vi "DB - [Setup].[Item] (Part Details).vi"(0 "connection reference":T14, 1 "DB Connection":T7={"Open"=TRUE, "Close"=TRUE}, 2 "DB - Setup Item Enum":T13=enum."INSERT [Setup].[Item]", 5 "DB.Schema.Table Array":string[](array[string]), 7 "Search Parameters":string, 9 "Transaction":T5, 11 "error in (no error)":errorcluster, 12 "DB Refnums":T6, 13 "OrderNo":string="101", 14 "DB Refnums II":T4) -> (3 "[IsMandatory] Ordered":string[](array[string]), 4 "connection reference":T14, 6 "1D Results":string[](array[string]), 8 "2D Results":string[][](array[string])=[["Production", "OperationNo1"], ["Production", "Qty1"], ["Production", "NCRNo1"], ["Production", "CustomerID1"], ["Production", "Customer1"], ["Production", "Project1"], ["Production", "SalesOrderNo1"], ["Production", "SalesOrderItemNo1"], ["Production", "MaterialNo1"], ["Production", "MaterialRev1"], ["Production", "MaterialDesc1"], ["Production", "SerialNos1"], ["Production", "UnitOfQty1"]], 10 "Transaction":T5, 15 "SUMMARY":errorcluster)   [LabVIEW 2020]
uses:
  <vilib>/addons/database/Connection.llb/Conn ObjectReference.ctl
  Control/DB - Setup Item Enum.ctl
  Control/Setup - Part Details - Item Details.ctl
  Control/Combo Box.ctl
  Control/DB - Logon Info.ctl
  Control/DB - OpenClose.ctl
  Control/DB - Refnums.ctl
  Control/Transaction Cluster.ctl
  Control/DB - Refnums II.ctl
  Control/Execute - Info.ctl
  Control/DB - [Setup].[Header] ColNames.ctl
  Control/DB - [TransactionNo],[OrderNo].ctl
  Variables/Global SRTRS.vi
  <vilib>/addons/database/Connection.llb/DB Tools Open Connec (String).vi
  <vilib>/addons/database/Connection.llb/Conn Execute.vi
  <vilib>/addons/database/Recordset.llb/Rec Fetch Recordset Data (R).vi
  <vilib>/addons/database/Recordset.llb/Rec Destroy - Connection.vi
  <vilib>/addons/database/Recordset.llb/Rec Fetch String Data (R).vi
  <vilib>/addons/database/_DB Variant To Data/Database Variant To Data.xnode
  <vilib>/addons/database/NI_Database_API.lvlib
panel:
  out "CASTed String":string
  out "SQL 1D Array":string[](array[string])
  in  "Results Output":cluster{"Output Set":T1, "Description":string}
  out "Ref error out":errorcluster={"status"=TRUE, "code"=1055, "source"="To More Specific Class in DB - Setup Item (Part Details).vi->Main.vi"}
  in  "Info. (Execute Tab)":T2 caption="Info." {"Variant Allowed (Hold Temp)" format="%.1f"}
  in  "CompactRIO Module Details":i32(listbox)=-1
  in  "Furnace Calibration":T3={"Furnace Serial No"="100", "Last Inspection Date"="2013-12-05", "Next Inspection Due Date"="2014-12-05"} caption="Furnace Details"
  out "Close Error":errorcluster
  out "Spreadsheet String":string[](array[string])
  in  "MCListBox FHS Setup":i32(listbox)=-1 caption="Furnace Heating Sequence"
  out "Refnums error out":errorcluster={"status"=TRUE, "code"=1055, "source"="To More Specific Class in DB - Setup Item (Part Details).vi->Main.vi"}
  in  "Part Details":i32(listbox)=-1
  in  "MCListBox AWPS":i32(listbox)=-1 caption="Additional WPS/Ref MCListBox"
  in  "Login":T8={"PlantID"="4070", "SystemID"="SRSB-2A", "UserID"="100001", "DomainID"="CCC", "LanguageID"="EN", "StationID"=""}
  in  "WPS Details Setup":T9={"WPS/Ref"="WPS5", "Rev"="1", "Hold Temperature"="100", "WPS Details Temperature Units"="°C", "Hold Time (HH:MM)"="1:00", "Inactive"=FALSE} caption="WPS Details"
  in  "Extra WPS":string caption="WPS"
  in  "Extra Rev":string caption="Rev."
  out "SQL 2D":string="Use [SRTRS]\n\nSELECT TOP 1 \n       [SourceTableName]\n      ,[SourceColumnName]\nFROM [Config].[Mapping]\nWHERE [TargetColumnName] = 'UnitOfQty'\n"
  in  "Channel Mapping":T10 caption="Channels Mapping"
  in  "Item Details":T11={"Order No."="102", "Oper. No."="102", "Qty."=1, "NCR No."="102", "NCR Boolean"=FALSE, "Customer No."="102", "Customer Name"="Cust102", "Project"="Proj102", "Sales Order"="SO102", "Item No."="SOI102", "Material"="M102", "Revision"="1", "Material Description"="", "Serial No."="102", "UnitOfQty"="Pallet"} {"Qty." min=1 max=99}
  in  "Notes":string="Hello World"
  in  "Plot":T12
  out "ms":u32
  out "Connection Information":T15={"Connection "="SQL Server 32bit HPEnvy", "Username"="admin", "Password"="admin123"}
  # "ONLY Witten to during LOGON (initialization)"
  # "For SELECT h.[TransactionNo], i.[OrderNo]\n\nSRTRS.Execute.Header\nSRTRS.Execute.Item\nSRTRS.MasterData.OutputSet"
  # "SRTRS.Setup.Header\nSRTRS.Setup.Item\nSRTRS.MasterData.OutputSet"
  # "Login\nItem Details\nWPS Details\nWPS (Extra)\nRev (Extra)\nAddtional WPS\nNotes\nParts Details (MCListBox)"
  # "[SourceTableName]        [SourceColumnName]           [IsMandatory]                 [TargetColumnName]"
  # "Column Hdrs[] are Important \nMust match with SRTRS Main.vi"
  # "Min"
  # "Min"
  # "Thermocouple"
  # "Probe No."
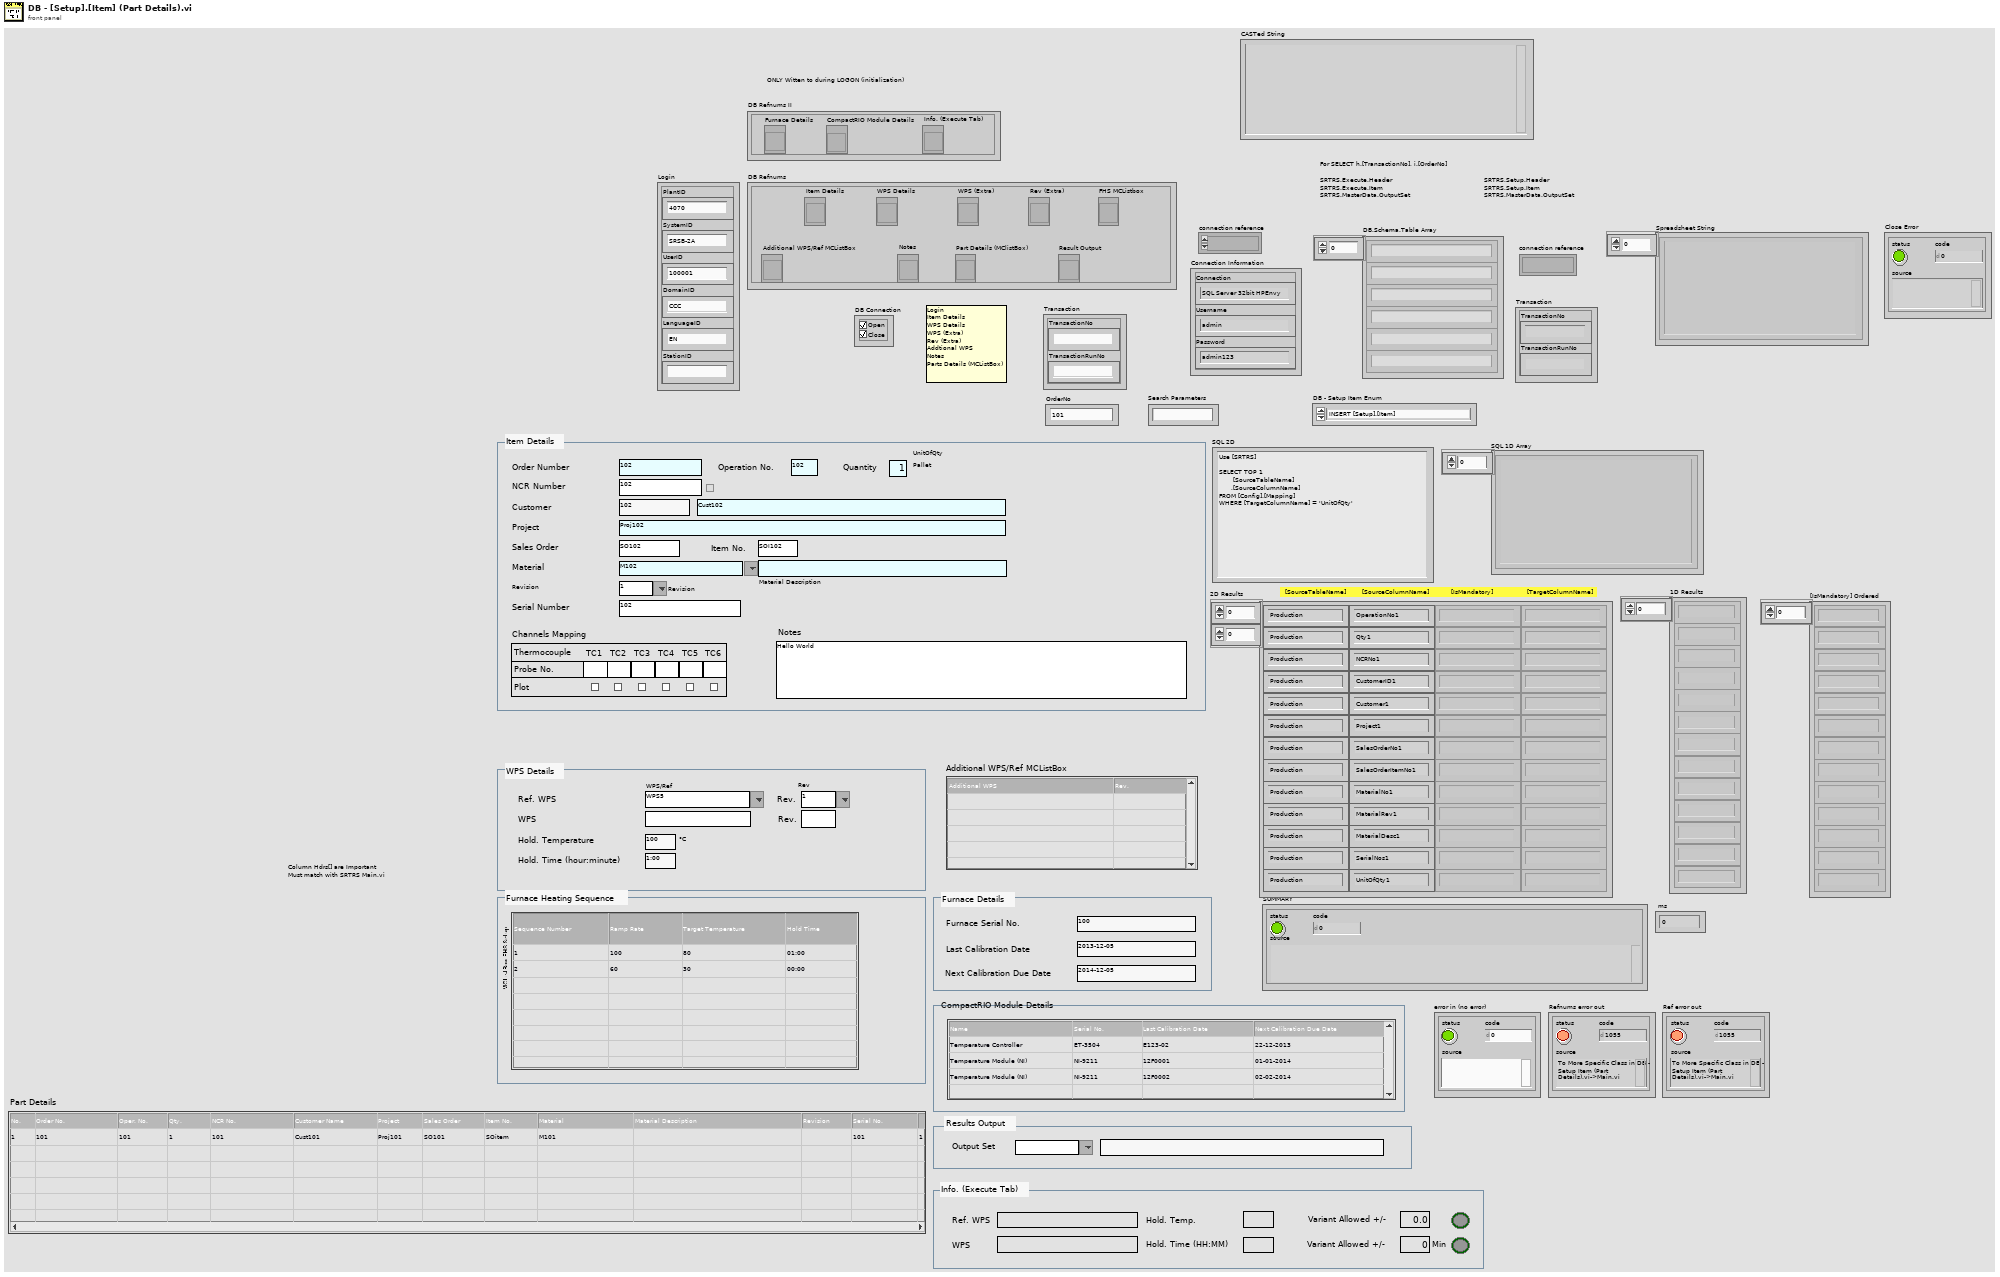
[diagram p1: front panel]
types:
  T1 = typedef "Combo Box.ctl" = string
  T2 = typedef "Execute - Info.ctl" = cluster{"Ref WPS":string, "Hold. Temp.":string, "Info. Temperature Units":string, "Variant Allowed (Hold Temp)":dbl, "Info. Temperature Units 2":string, "Variant Allowed (Hold Temp)":bool, "Hold. Time (hour:minute)":string, "Variant Allowed (Hold Time)":dbl, "Variant Allowed (Hold Time)":bool, "WPS":string}
  T3 = cluster{"Furnace Serial No":string, "Last Inspection Date":string, "Next Inspection Due Date":string}
  T4 = typedef "DB - Refnums II.ctl" = cluster{"Furnace Details":refnum<vi>, "CompactRIO Module Details":refnum<vi>, "Info. (Execute Tab)":refnum<vi>}
  T5 = typedef "Transaction Cluster.ctl" = cluster{"TransactionNo":string, "TransactionRunNo":string}
  T6 = typedef "DB - Refnums.ctl" = cluster{"Item Details":refnum<vi>, "WPS Details":refnum<vi>, "WPS (Extra)":refnum<vi>, "Rev (Extra) ":refnum<vi>, "FHS MCListbox":refnum<vi>, "Additional WPS/Ref MCListBox":refnum<vi>, "Notes":refnum<vi>, "Part Details (MClistBox)":refnum<vi>, "Result Output":refnum<vi>}
  T7 = typedef "DB - OpenClose.ctl" = cluster{"Open":bool, "Close":bool}
  T8 = typedef "DB - Logon Info.ctl" = cluster{"PlantID":string, "SystemID":string, "UserID":string, "DomainID":string, "LanguageID":string, "StationID":string}
  T9 = cluster{"WPS/Ref":T1, "Rev":T1, "Hold Temperature":string, "WPS Details Temperature Units":string, "Hold Time (HH:MM)":string, "Inactive":bool}
  T10 = cluster{"TC1":string, "TC2":string, "TC3":string, "TC4":string, "TC5":string, "TC6":string}
  T11 = typedef "Setup - Part Details - Item Details.ctl" = cluster{"Order No.":string, "Oper. No.":string, "Qty.":i32, "NCR No.":string, "NCR Boolean":bool, "Customer No.":string, "Customer Name":string, "Project":string, "Sales Order":string, "Item No.":string, "Material":string, "Revision":string, "Material Description":string, "Serial No.":string, "UnitOfQty":string}
  T12 = cluster{"TC01Plot":bool, "TC02Plot":bool, "TC03Plot":bool, "TC04Plot":bool, "TC05Plot":bool, "TC06Plot":bool}
  T13 = typedef "DB - Setup Item Enum.ctl" = enum16{"SELECT [Plant],[OrderNo]", "INSERT [Setup].[Header]", "INSERT [Setup].[Item]", "INSERT [Setup].[ProcedureItem]", "SELECT [TransactionNo]", "SELECT [TransactionNo], others", "SELECT [OrderNo]", "SELECT [OrderNo], others", "SELECT h.[TransactionNo], i.[OrderNo]", "SELECT [Setup].[ProcedureItem]", "SELECT [EquipmentxId]"}
  T14 = typedef "NI_Database_API.lvlib/Conn ObjectReference.ctl" = refnum<k1>
  T15 = cluster{"Connection ":string, "Username":string, "Password":string}
  T16 = typedef "Enum - InteractiveMode-SubVIMode.ctl" = enum16{"Interactive", "subVI Mode"}
  T17 = typedef "Connection Information Cluster.ctl" = cluster{"Connection ":string, "Username":string, "Password":string}
  T18 = typedef "DB - DB.Schema.Table.ctl" = cluster{"DB":string, "Schema":string, "Table":string}
  T19 = typedef "DB - [TransactionNo],[OrderNo].ctl" = enum16{"h.[TransactionNo]", "h.[ProcedureNo]", "h.[ProcedureRev]", "h.[WPSNo]", "h.[WPSRev]", "h.[HoldTemperature]", "h.[UnitOfTemperature]", "h.[HoldTime]", "h.[AdditionalProcs]", "h.[OutputSetId]", "h.[PermittedTempDiff]", "h.[PermittedTimeDiff]", "j.[Description]", "i.[itemNo]", "i.[OrderNo]", "i.[OperationNo]", "i.[Qty]", "i.[UnitOfQty]", "i.[NCRIndicator]", "i.[NCRNo]", "i.[CustomerID]", "i.[Customer]", "i.[Project]", "i.[SalesOrderNo]", "i.[SalesOrderItemNo]", "i.[MaterialNo]", "i.[MaterialDesc]", "i.[MaterialRev]", "i.[SerialNos]", "i.[Notes]", "i.[TC01]", "i.[TC02]", "i.[TC03]", "i.[TC04]", "i.[TC05]", "i.[TC06]", "i.[TC01Plot]", "i.[TC02Plot]", "i.[TC03Plot]", "i.[TC04Plot]", "i.[TC05Plot]", "i.[TC06Plot]"}
  T20 = typedef "NI_Database_API.lvlib/Rec ObjectReference.ctl" = refnum<k1>
  T21 = typedef "DB - Logon Extra Info.ctl" = cluster{"Plant Name":string, "UserName":string, "Hostname [ClientName]":string, "IsUnicode":bool}
  T22 = typedef "DB - [Setup].[Header] ColNames.ctl" = enum16{"[TransactionNo]", "[PlantID]", "[SystemID]", "[ProcedureNo]", "[ProcedureRev]", "[WPSNo]", "[WPSRev]", "[HoldTemperature]", "[UnitOfTemperature]", "[HoldTime]", "[AdditionalProcs]", "[OutputSetId]", "[Equipment1ID]", "[Equipment2ID]", "[Equipment3ID]", "[Equipment4ID]", "[Equipment5ID]", "[Equipment6ID]", "[Equipment7ID]", "[Equipment8ID]", "[Equipment9ID]", "[Equipment10ID]", "[PermittedTempDiff]", "[PermittedTimeDiff]", "[Notes]", "[CreatedBy]", "[CreatedOn]", "[LastSavedBy]", "[LastSavedOn]"}
  T23 = cluster{"TransactionNo":string, "TransactionRunNo":string}
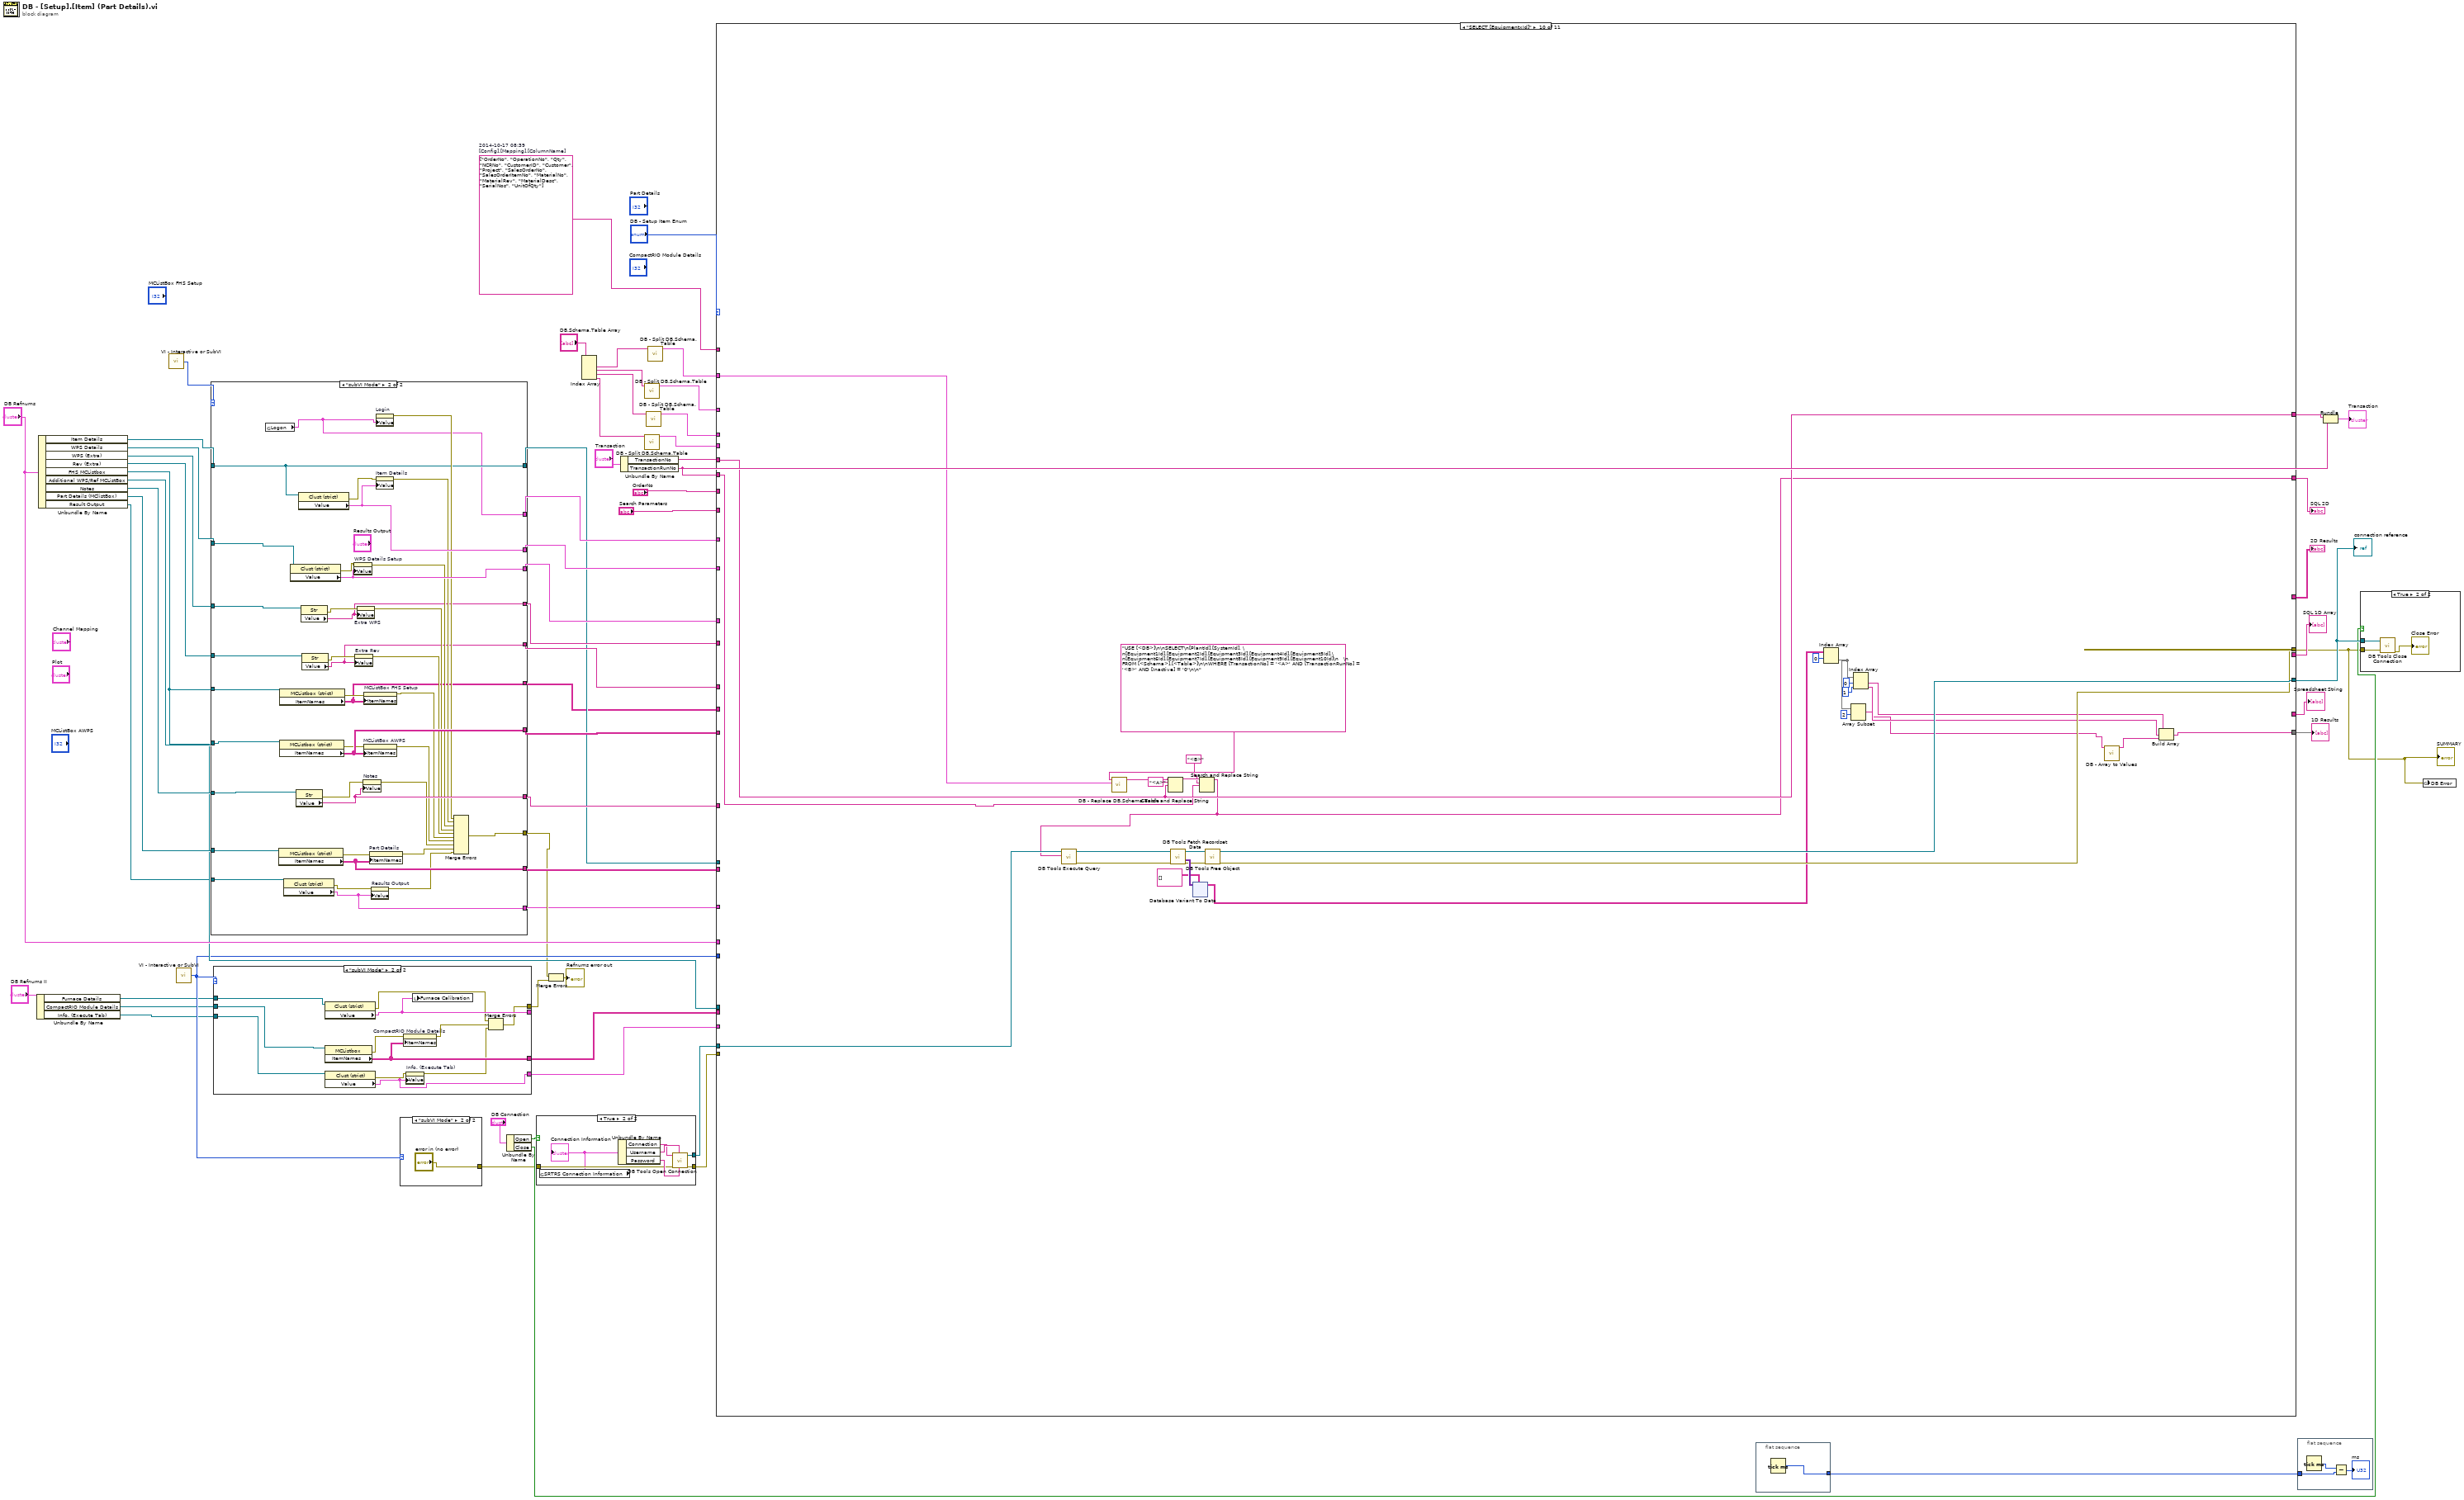
[diagram p0: block diagram]
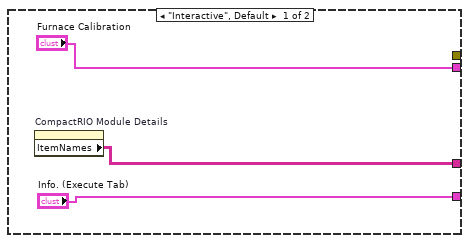
[diagram p2: hidden frame]
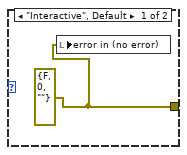
[diagram p3: hidden frame]
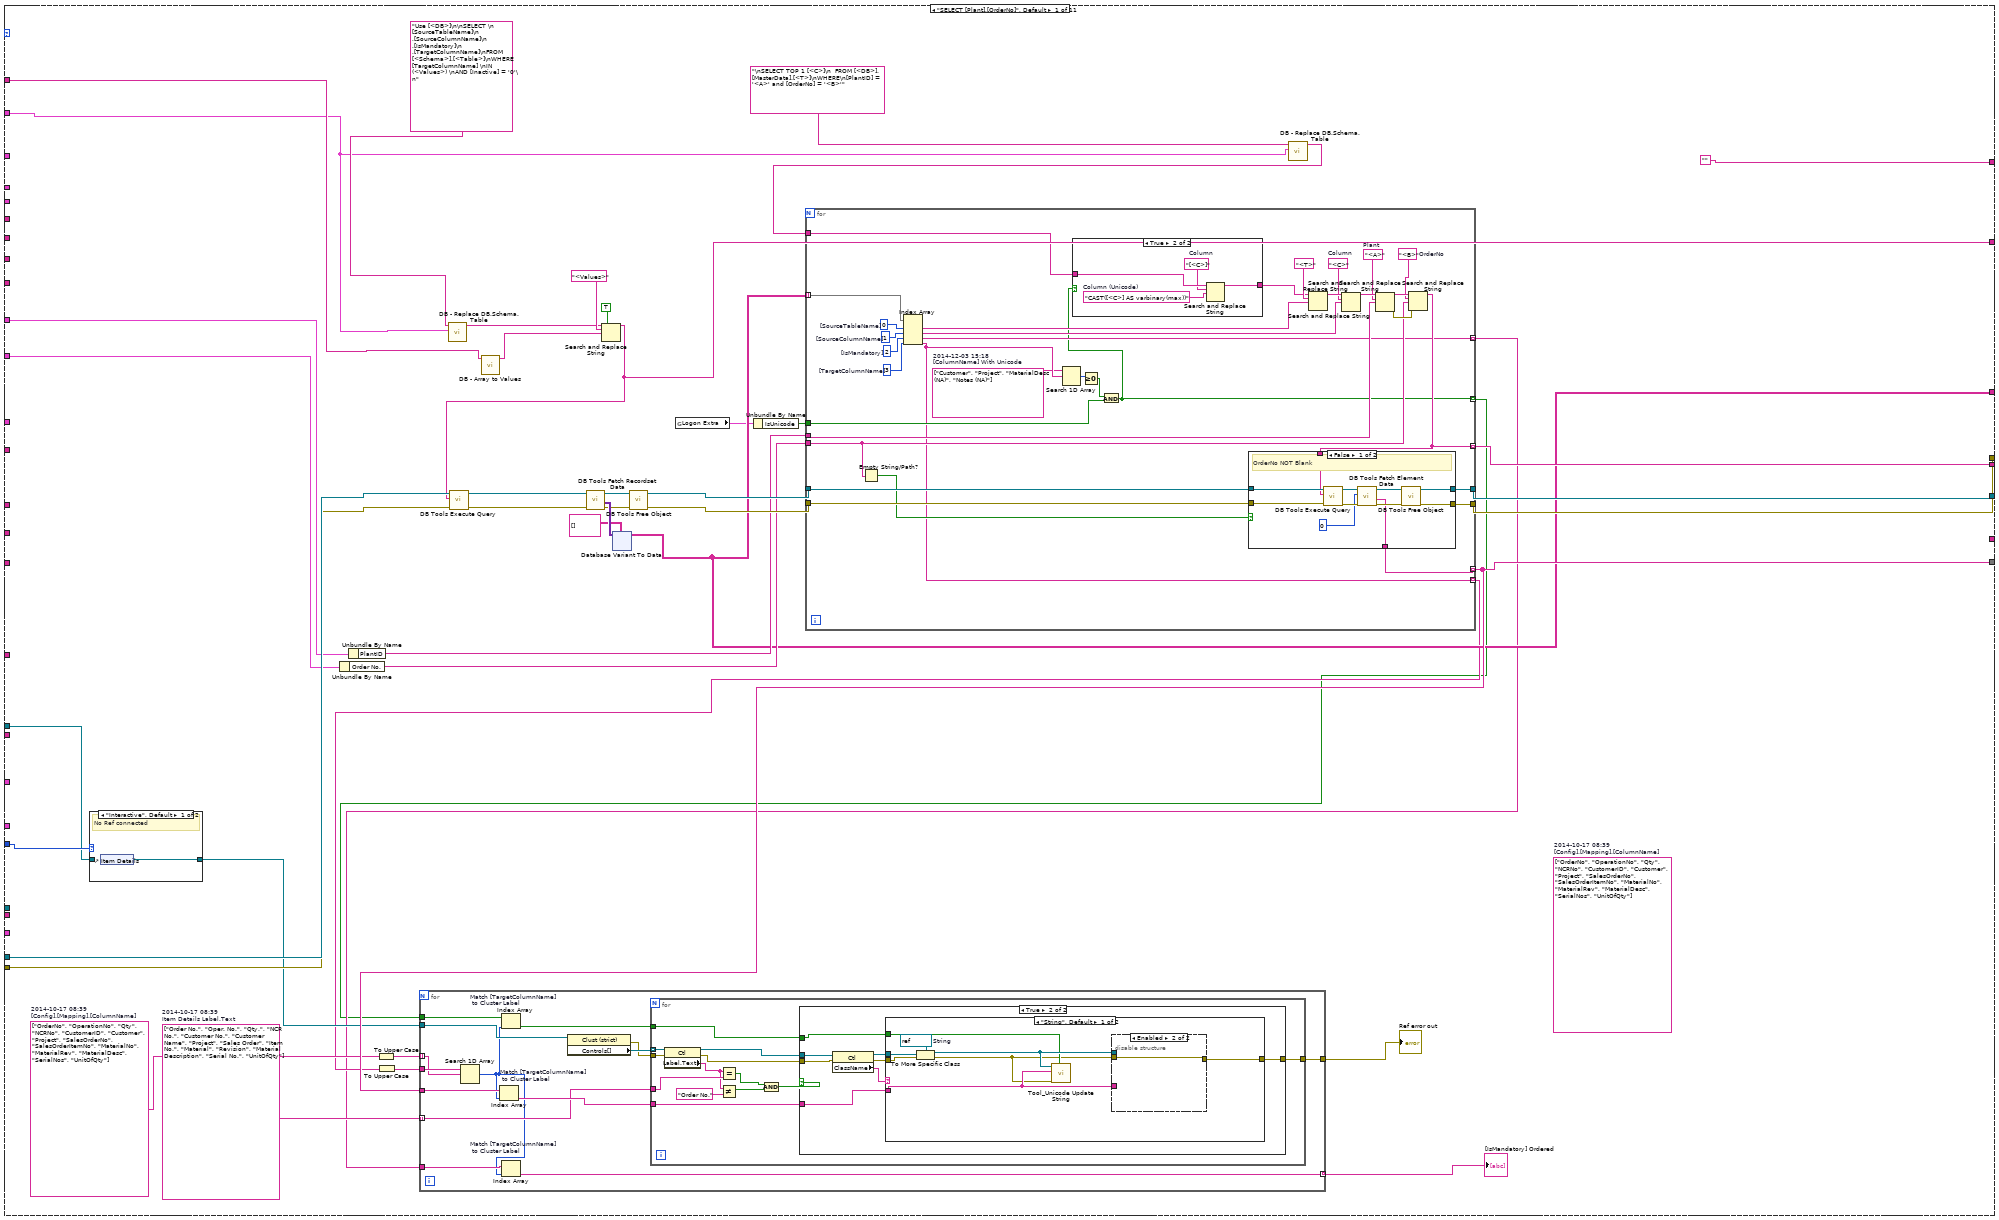
[diagram p4: hidden frame]
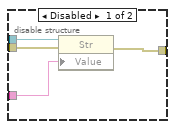
[diagram p6: hidden frame]
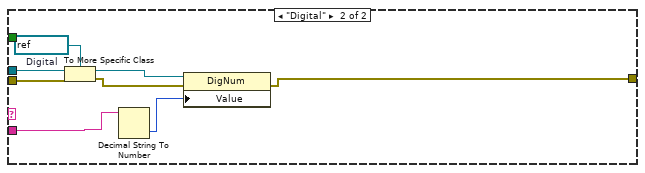
[diagram p7: hidden frame]
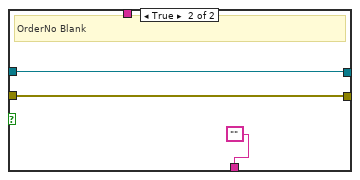
[diagram p10: hidden frame]
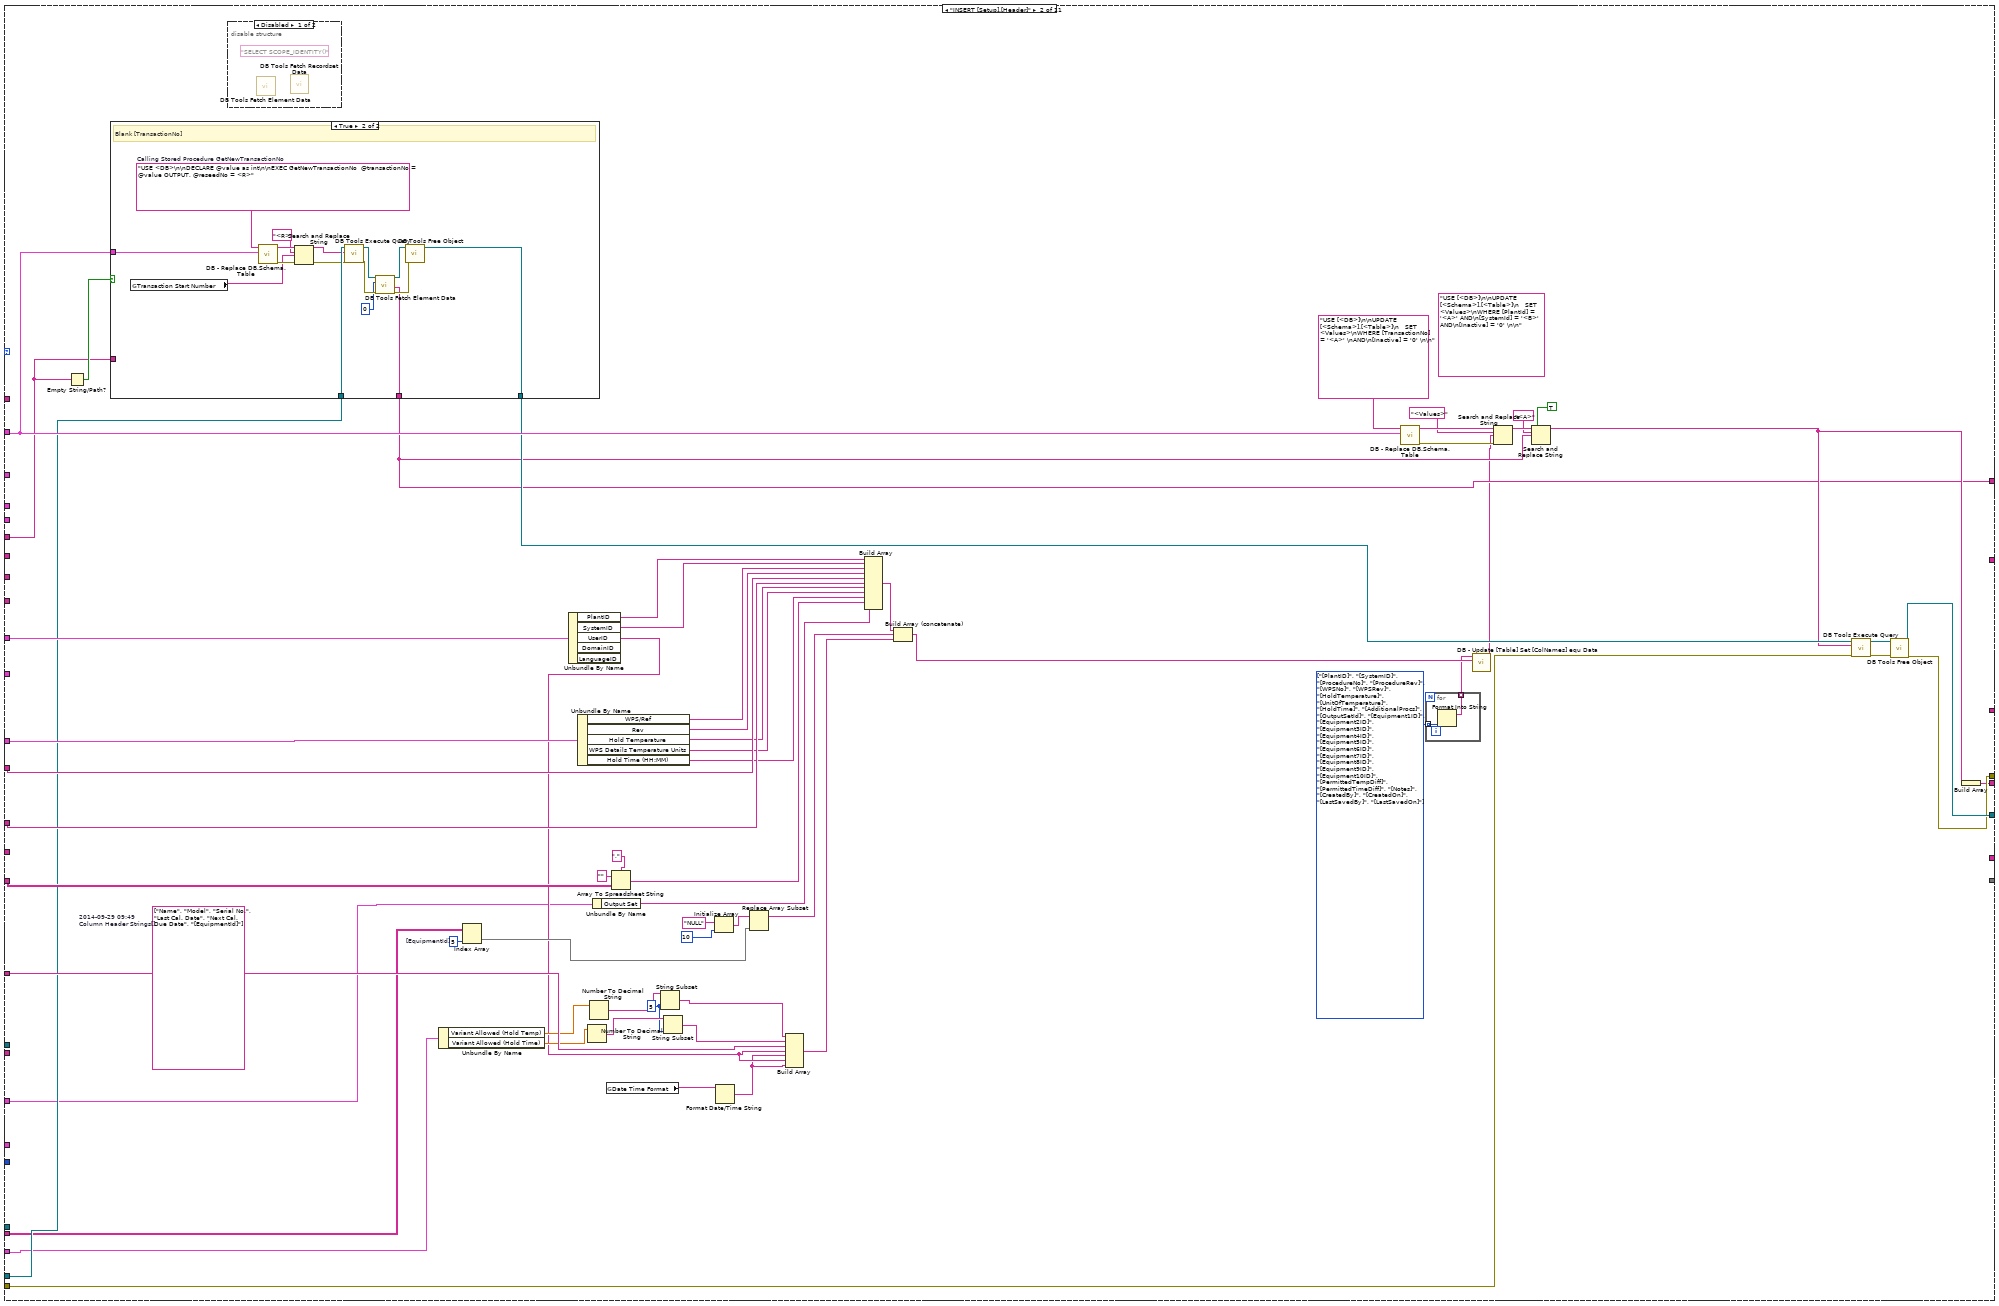
[diagram p11: hidden frame]
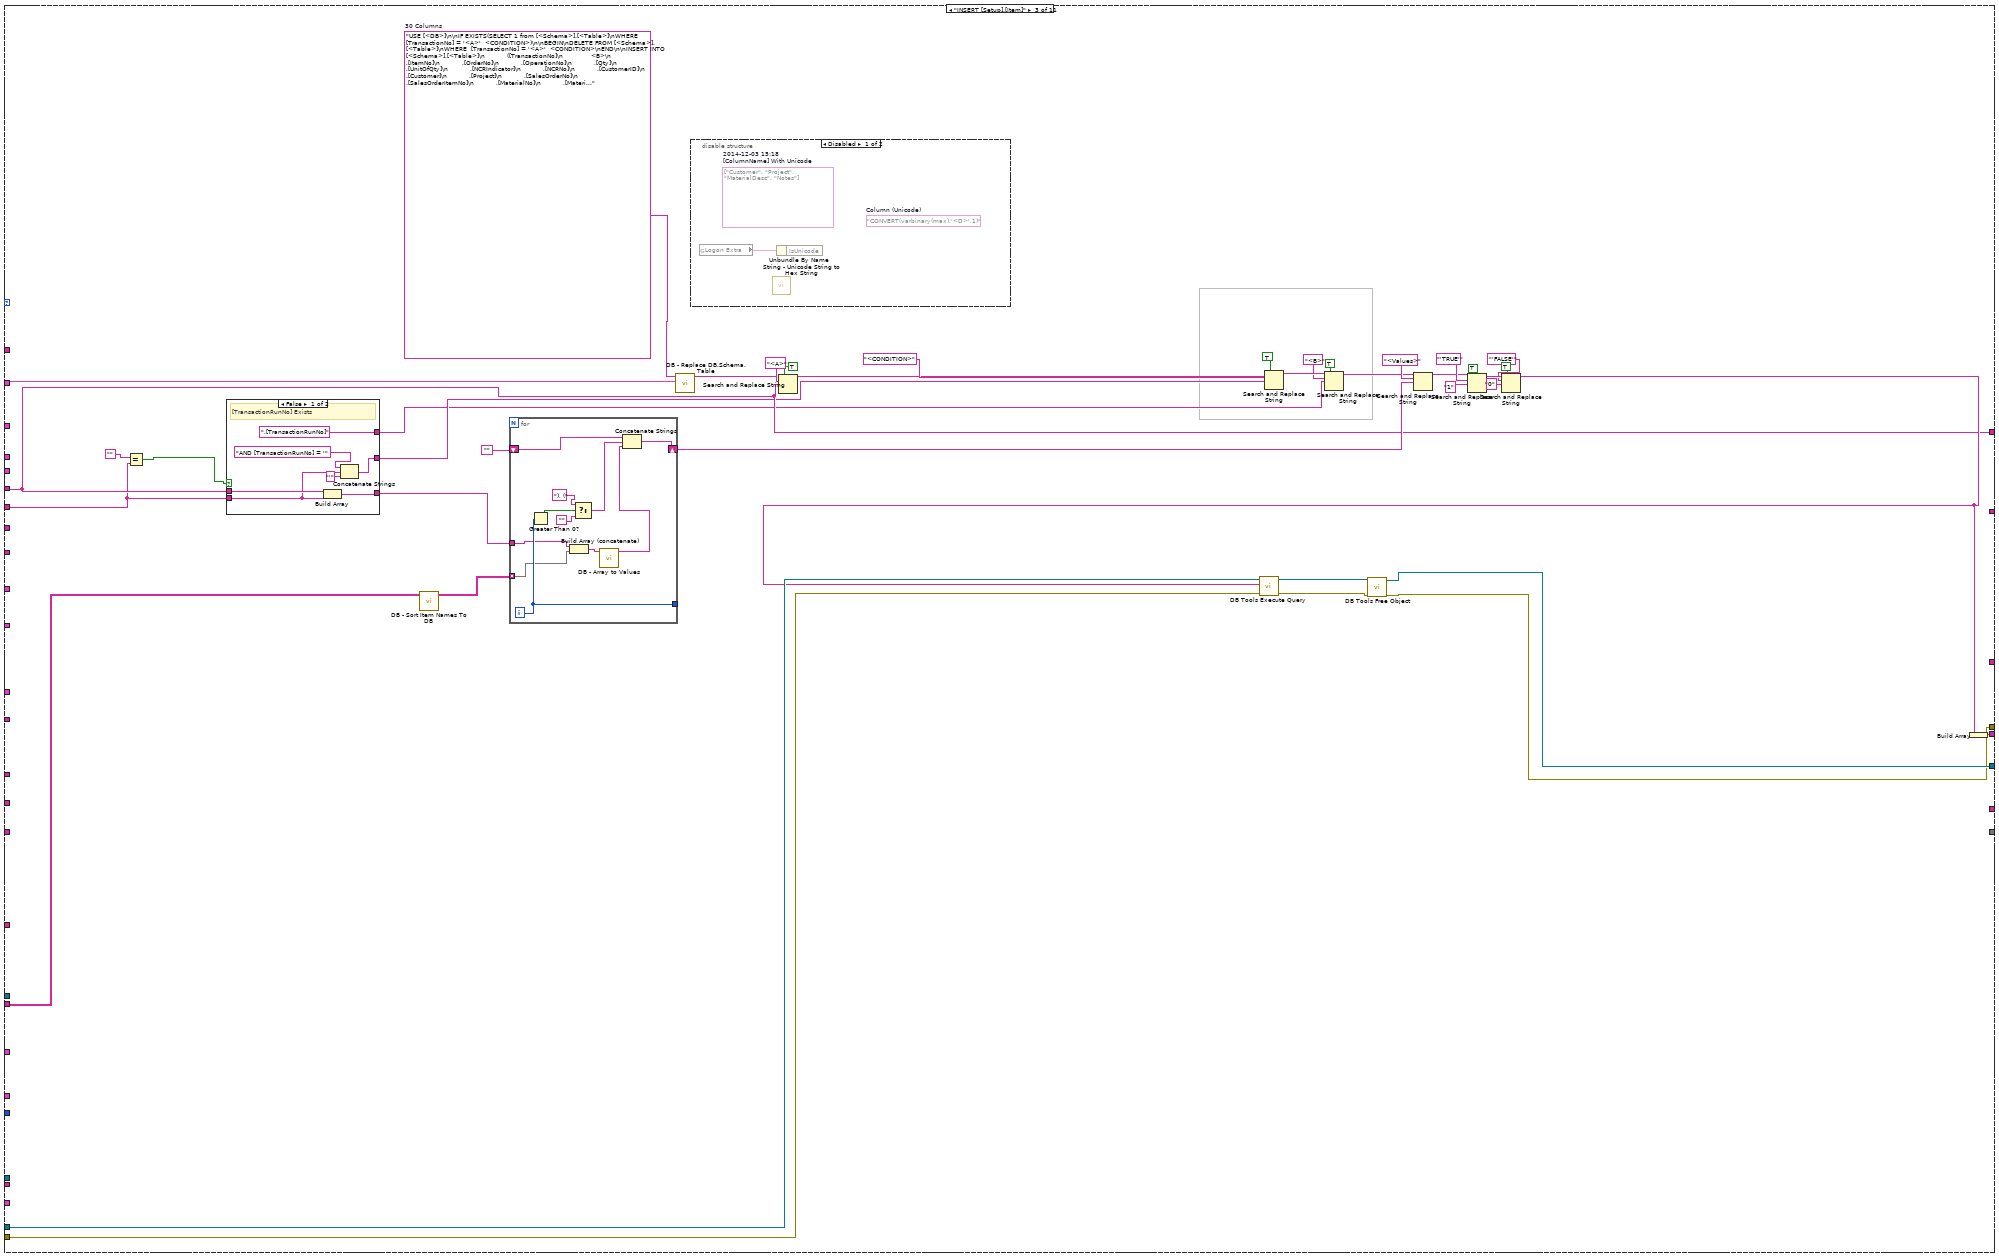
[diagram p14: hidden frame]
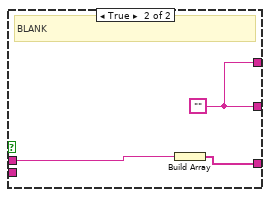
[diagram p16: hidden frame]
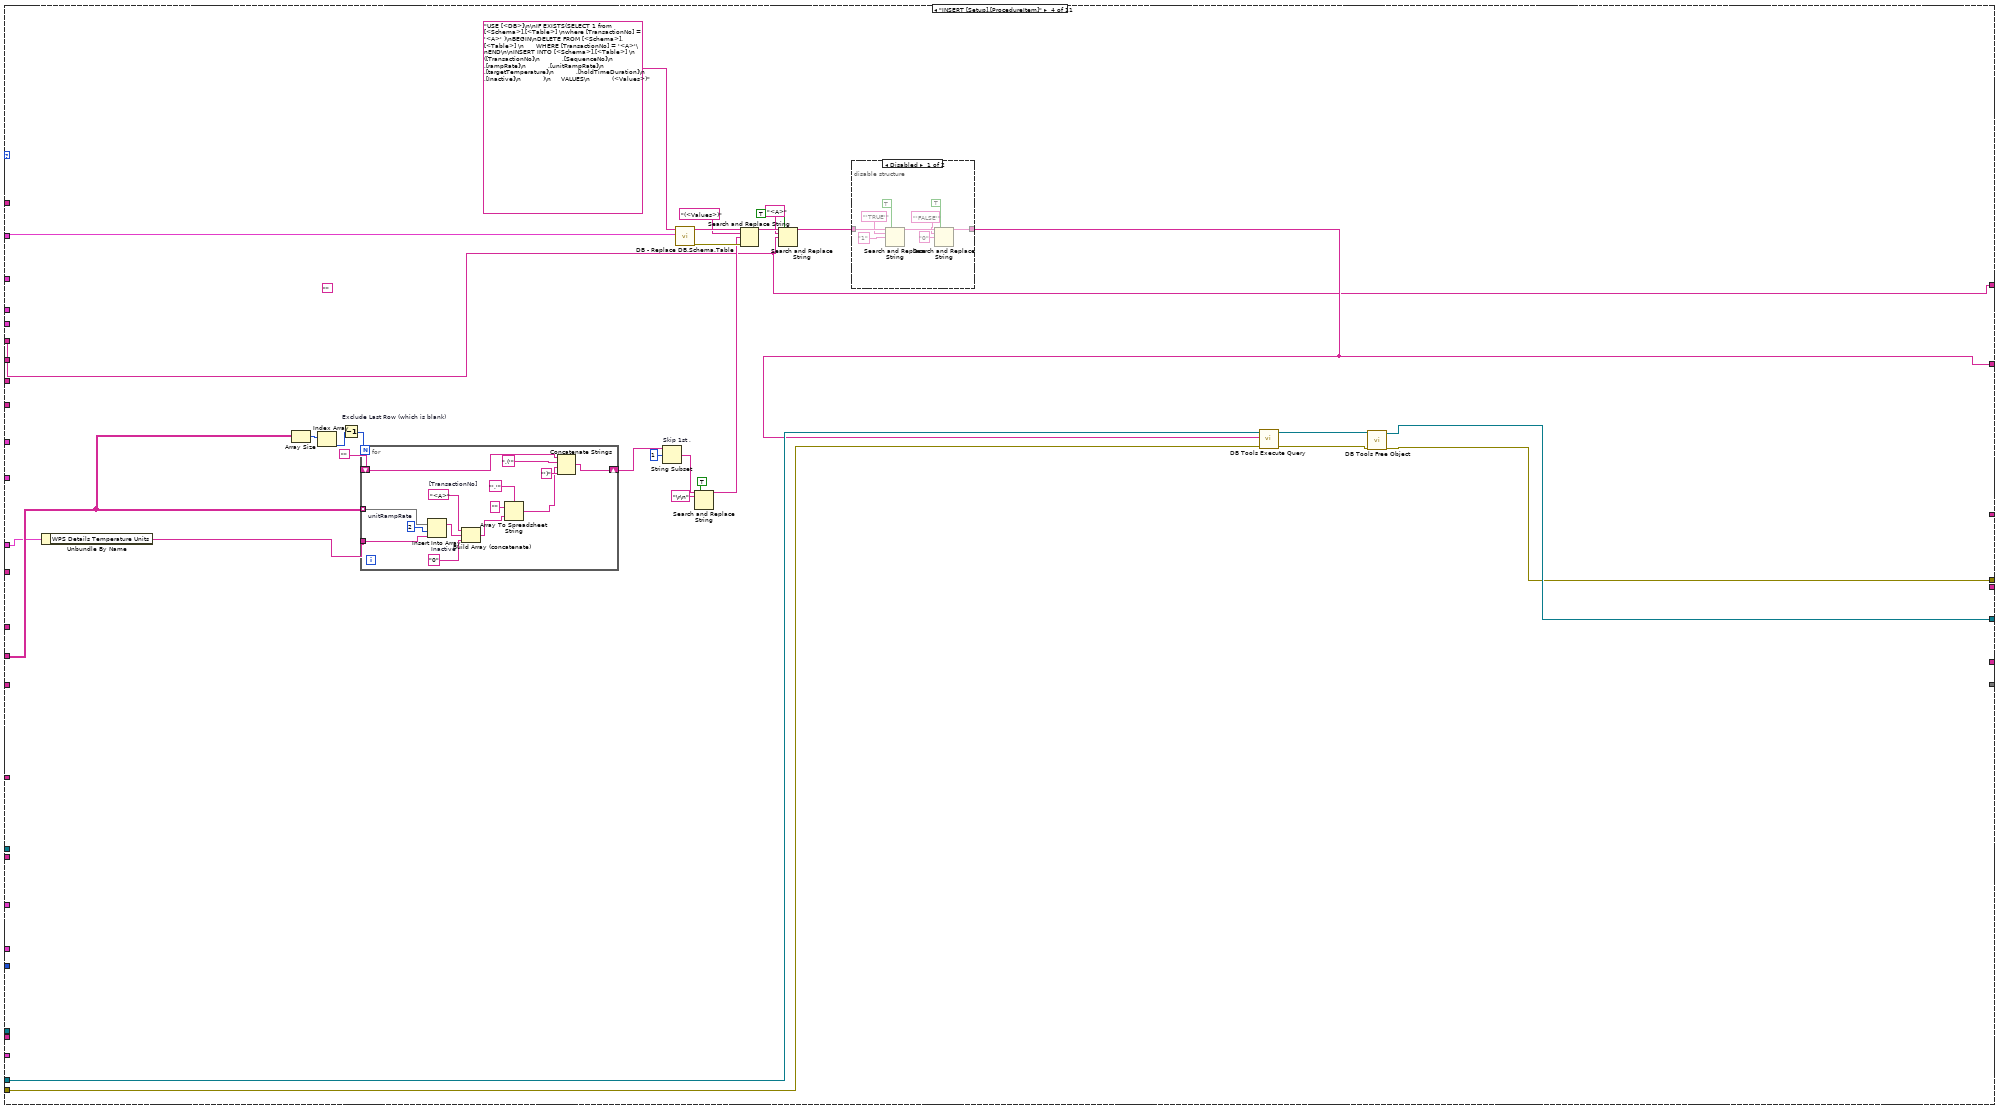
[diagram p17: hidden frame]
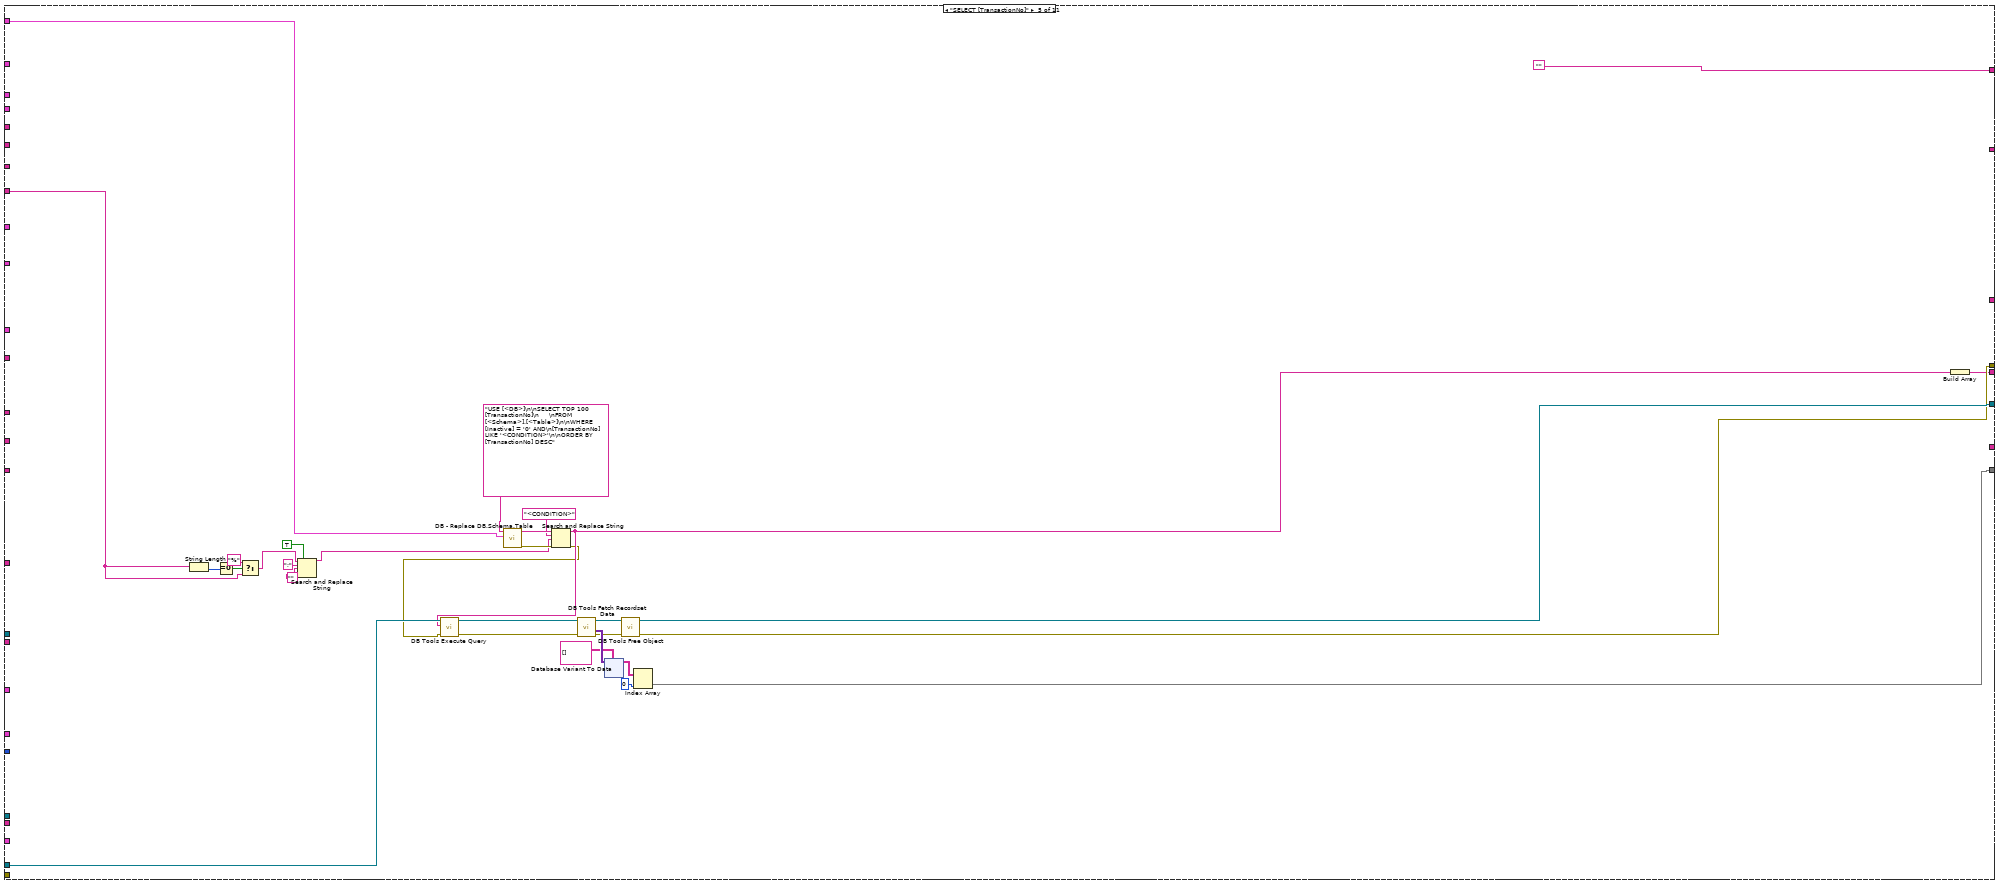
[diagram p19: hidden frame]
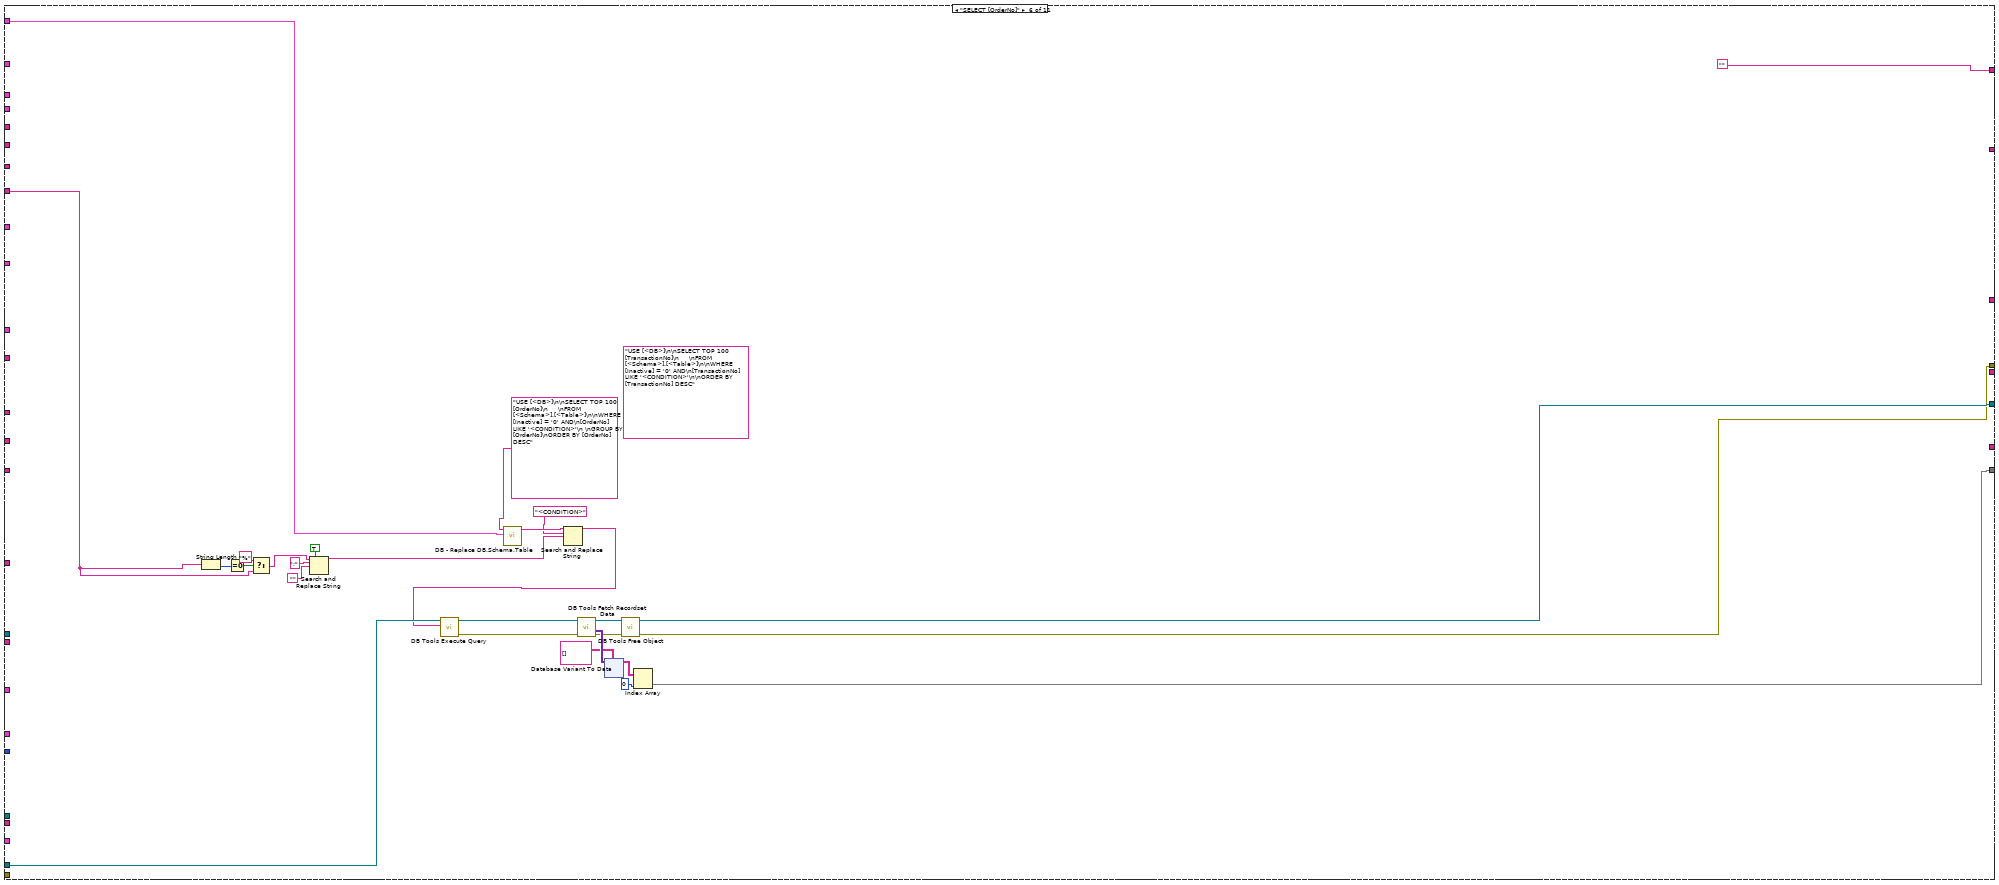
[diagram p20: hidden frame]
diagram:
  w1 = string[] ["OrderNo", "OperationNo", "Qty", "NCRNo", "CustomerID", "Customer", "Project", "SalesOrderNo", "SalesOrderItemNo", "MaterialNo", "MaterialRev", "MaterialDesc", "SerialNos", "UnitOfQty"]  # 2014-10-17 08:39 [Config].[Mapping].[ColumnName]
  n1 = Unbundle By Name("DB Refnums II") -> ("Furnace Details"=w11:refnum<vi>, "CompactRIO Module Details"=w10:refnum<vi>, "Info. (Execute Tab)"=w5:refnum<vi>)
  n2 = Unbundle By Name("DB Refnums") -> ("Item Details"=w45:refnum<vi>, "WPS Details"=w44:refnum<vi>, "WPS (Extra)"=w43:refnum<vi>, "Rev (Extra)"=w42:refnum<vi>, "FHS MCListbox"=w32:refnum<vi>, "Additional WPS/Ref MCListBox"=w41:refnum<vi>, "Notes"=w40:refnum<vi>, "Part Details (MClistBox)"=w39:refnum<vi>, "Result Output"=w3:refnum<vi>)
  n3 = call "VI - Interactive or SubVI.vi"() -> ("Mode"=w14:T16)  [unwired: 5 in]
  n4 = call "VI - Interactive or SubVI.vi"() -> ("Mode"=w13:T16)  [unwired: 5 in]
  n5 = case shown="\"subVI Mode\"" w14 {
    tunnel: ["Item Details" w113] -> w52
    tunnel: ["Login" w79] -> w54
    tunnel: ["WPS Details Setup" w112] -> w53
    tunnel: ["Extra Rev" w86] -> w51
    tunnel: ["Extra WPS" w85] -> w50
    tunnel: w41 -> [_ w89]
    tunnel: [w71 w111] -> w49
    tunnel: ["Notes" w103] -> w48
    tunnel: w45 -> [_ w93]
    tunnel: w43 -> [_ w91]
    tunnel: w40 -> [_ w88]
    tunnel: [_ w93] -> w47
    tunnel: w39 -> [_ w87]
    tunnel: [w67 w110] -> w46
    tunnel: w44 -> [_ w92]
    tunnel: w42 -> [_ w90]
    tunnel: w32 -> [_ w84]
    tunnel: [w66 w81] -> w33
    tunnel: [_ w80] -> w9
    tunnel: w3 -> [_ w78]
    tunnel: [w65 w75] -> w2
    frame "Interactive", Default {
      n6 = property on="MCListBox FHS Setup" class="MCListbox (strict)"() -> ("ItemNames"=w66:string[][])  [unwired: 2 in, 2 out]
      n7 = property on="Part Details" class="MCListbox (strict)"() -> ("ItemNames"=w67:string[][])  [unwired: 2 in, 2 out]
      n8 = property on="MCListBox AWPS" class="MCListbox (strict)"() -> ("ItemNames"=w71:string[][])  [unwired: 2 in, 2 out]
      n9 = property on="Results Output" class="Clust (strict)"() -> ("Value"=w65:cluster{"Output Set":T1, "Description":string})  [unwired: 2 in, 2 out]
    }
    frame "subVI Mode" {
      n10 = global read "Global SRTRS.vi" "Logon"() -> (w79:T8)
      n11 = property class="MCListbox (strict)"(reference=w87) -> (error out=w94:errorcluster, "ItemNames"=w110:string[][])  [unwired: 1 in, 1 out]
      n12 = property class="MCListbox (strict)"(reference=w89) -> (error out=w105:errorcluster, "ItemNames"=w111:string[][])  [unwired: 1 in, 1 out]
      n13 = property class="MCListbox (strict)"(reference=w84) -> (error out=w83:errorcluster, "ItemNames"=w81:string[][])  [unwired: 1 in, 1 out]
      n14 = property class="Clust (strict)"(reference=w78) -> (error out=w77:errorcluster, "Value"=w75:cluster{"Output Set":T1, "Description":string})  [unwired: 1 in, 1 out]
      n15 = property class="Clust (strict)"(reference=w92) -> (error out=w108:errorcluster, "Value"=w112:T9)  [unwired: 1 in, 1 out]
      n16 = property class="Str"(reference=w88) -> (error out=w104:errorcluster, "Value"=w103:string)  [unwired: 1 in, 1 out]
      n17 = property class="Clust (strict)"(reference=w93) -> (error out=w109:errorcluster, "Value"=w113:T11)  [unwired: 1 in, 1 out]
      n18 = property class="Str"(reference=w91) -> (error out=w107:errorcluster, "Value"=w86:string)  [unwired: 1 in, 1 out]
      n19 = property class="Str"(reference=w90) -> (error out=w106:errorcluster, "Value"=w85:string)  [unwired: 1 in, 1 out]
      n20 = property on="WPS Details Setup" class="Clust (strict)"(error in=w108, "Value"=w112) -> (error out=w100:errorcluster)  [unwired: 1 in, 1 out]
      n21 = property on="Extra Rev" class="Str"(error in=w106, "Value"=w85) -> (error out=w98:errorcluster)  [unwired: 1 in, 1 out]
      n22 = property on="Extra WPS" class="Str"(error in=w107, "Value"=w86) -> (error out=w99:errorcluster)  [unwired: 1 in, 1 out]
      n23 = property on="Notes" class="Str"(error in=w104, "Value"=w103) -> (error out=w96:errorcluster)  [unwired: 1 in, 1 out]
      n24 = property on="MCListBox AWPS" class="MCListbox (strict)"(error in=w105, "ItemNames"=w111) -> (error out=w97:errorcluster)  [unwired: 1 in, 1 out]
      n25 = property on="MCListBox FHS Setup" class="MCListbox (strict)"(error in=w83, "ItemNames"=w81) -> (error out=w82:errorcluster)  [unwired: 1 in, 1 out]
      n26 = property on="Part Details" class="MCListbox (strict)"(error in=w94, "ItemNames"=w110) -> (error out=w95:errorcluster)  [unwired: 1 in, 1 out]
      n27 = property on="Results Output" class="Clust (strict)"(error in=w77, "Value"=w75) -> (error out=w76:errorcluster)  [unwired: 1 in, 1 out]
      n28 = property on="Login" class="Clust (strict)"("Value"=w79) -> (error out=w102:errorcluster)  [unwired: 2 in, 1 out]
      n29 = property on="Item Details" class="Clust (strict)"(error in=w109, "Value"=w113) -> (error out=w101:errorcluster)  [unwired: 1 in, 1 out]
      n30 = Merge Errors(w102, w101, w100, w99, w98, w82, w97, w96, w95, w76) -> (w80:errorcluster)
    }
  }
  n31 = case shown="\"subVI Mode\"" w13 {
    tunnel: w11 -> [_ w128]
    tunnel: w10 -> [_ w127]
    tunnel: ["Furnace Calibration" w124] -> _
    tunnel: [w115 w125] -> w6
    tunnel: [_ w121] -> w8
    tunnel: ["Info. (Execute Tab)" w117] -> w4
    tunnel: w5 -> [_ w120]
    frame "Interactive", Default {
      n32 = property on="CompactRIO Module Details" class="MCListbox (strict)"() -> ("ItemNames"=w115:string[][])  [unwired: 2 in, 2 out]
    }
    frame "subVI Mode" {
      n33 = property class="Clust (strict)"(reference=w128) -> (error out=w123:errorcluster, "Value"=w124:T3)  [unwired: 1 in, 1 out]
      n34 = property class="MCListbox"(reference=w127) -> (error out=w126:errorcluster, "ItemNames"=w125:string[][])  [unwired: 1 in, 1 out]
      n35 = property class="Clust (strict)"(reference=w120) -> (error out=w119:errorcluster, "Value"=w117:T2)  [unwired: 1 in, 1 out]
      n36 = property on="CompactRIO Module Details" class="MCListbox (strict)"(error in=w126, "ItemNames"=w125) -> (error out=w122:errorcluster)  [unwired: 1 in, 1 out]
      n37 = property on="Info. (Execute Tab)" class="Clust (strict)"(error in=w119, "Value"=w117) -> (error out=w118:errorcluster)  [unwired: 1 in, 1 out]
      n38 = local write "Furnace Calibration"(w124) -> ()
      n39 = Merge Errors(w123, w122, w118) -> (w121:errorcluster)
    }
  }
  n40 = case shown="\"subVI Mode\"" w13 {
    tunnel: [w129 "error in (no error)"] -> w36
    frame "Interactive", Default {
      w129 = errorcluster {"status"=FALSE, "code"=0, "source"=""} ("error in (no error)")
      n41 = local write "error in (no error)"(w129) -> ()
    }
    frame "subVI Mode" {
    }
  }
  n42 = Unbundle By Name("DB Connection") -> ("Open"=w56:bool, "Close"=w55:bool)
  n43 = case shown="True" w56 {
    tunnel: ["connection reference" w136] -> w16
    tunnel: w36 -> [w131 w135]
    tunnel: [w131 w134] -> w15
    frame False {
      # "subVI"
    }
    frame True {
      n44 = global read "Global SRTRS.vi" "SRTRS Connection Information"() -> (w133:T17)
      "Connection Information" <- w133
      n45 = Unbundle By Name(w133) -> ("Connection"=w138:string, "Username"=w139:string, "Password"=w137:string)
      n46 = call-poly <vilib>:"DB Tools Open Connection.vi"("password"=w137, "userID"=w139, "error in (no error)"=w135, "connection information"=w138) -> ("error out"=w134:errorcluster, "connection reference"=w136:T14)  [unwired: 4 in]
    }
  }
  n47 = Merge Errors(w9, w8) -> (→"Refnums error out":errorcluster)
  n48 = Index Array(array="DB.Schema.Table Array") -> (element #1=w21:string, element #2=w20:string, element #3=w19:string, element #4=w18:string)  [unwired: 4 in]
  n49 = Unbundle By Name("Transaction") -> ("TransactionNo"=w28:string, "TransactionRunNo"=w25:string)
  n50 = call "DB - Split DB.Schema.Table.vi"("DB.Schema.Table"=w20) -> ("DB.Schema.Table"=w60:T18)  [unwired: 10 in]
  n51 = call "DB - Split DB.Schema.Table.vi"("DB.Schema.Table"=w18) -> ("DB.Schema.Table"=w17:T18)  [unwired: 10 in]
  n52 = call "DB - Split DB.Schema.Table.vi"("DB.Schema.Table"=w19) -> ("DB.Schema.Table"=w31:T18)  [unwired: 10 in]
  n53 = call "DB - Split DB.Schema.Table.vi"("DB.Schema.Table"=w21) -> ("DB.Schema.Table"=w64:T18)  [unwired: 10 in]
  n54 = case shown="\"SELECT [EquipmentxId]\"" "DB - Setup Item Enum" {
    tunnel: w16 -> [w183 w364 w457 w507 w556 w627 w692 w758 w837 w919 w1053]
    tunnel: [w175 w368 w455 w505 w555 w626 w691 w757 w836 w918 w1052] -> w58
    tunnel: [w176 w367 w454 w504 w554 w625 w690 w756 w835 w917 w1013] -> w23
    tunnel: w64 -> [w150 w365 w459 w511 w558 w629 w694 w759 w839 w921 w1054]
    tunnel: [w174 w338 w421 _ w536 _ _ _ _ _ _] -> w59
    tunnel: w15 -> [w182 w376 w456 w506 _ _ _ _ _ _ _]
    tunnel: [w166 _ _ _ w553 w624 _ _ _ w907 _] -> w61
    tunnel: w47 -> [w165 _ _ _ _ _ _ _ _ _ _]
    tunnel: w60 -> [_ _ _ _ _ _ w688 w754 _ _ w1049]
    tunnel: w1 -> [w154 _ _ _ _ _ _ _ _ _ _]
    tunnel: w54 -> [w171 w396 _ _ _ _ _ _ _ _ _]
    tunnel: w53 -> [_ w395 _ w484 _ _ _ _ _ _ _]
    tunnel: w52 -> [w173 _ _ _ _ _ _ _ _ _ _]
    tunnel: w51 -> [_ w392 _ _ _ _ _ _ _ _ _]
    tunnel: w50 -> [_ w391 _ _ _ _ _ _ _ _ _]
    tunnel: w49 -> [_ w387 _ _ _ _ _ _ _ _ _]
    tunnel: w48 -> [_ w377 _ _ _ _ _ _ _ _ _]
    tunnel: w13 -> [w169 _ _ _ _ _ _ _ _ _ _]
    tunnel: w28 -> [_ w362 w427 w482 _ _ w683 _ w826 w914 w1011]
    tunnel: w46 -> [_ _ w452 _ _ _ _ _ _ _ _]
    tunnel: [w168 _ _ w496 _ _ w685 w751 w817 w912 w1010] -> w38
    tunnel: [w152 _ _ _ _ _ w686 w752 w812 _ w985] -> w37
    tunnel: "OrderNo" -> [_ _ _ _ _ _ _ w750 _ _ _]
    tunnel: "DB Refnums" -> [_ _ _ _ _ _ _ _ _ _ w1046]
    tunnel: w33 -> [_ _ _ w485 _ _ _ _ _ _ _]
    tunnel: w32 -> [_ _ _ _ _ _ _ _ w833 _ _]
    tunnel: w31 -> [_ _ _ _ _ _ w684 w749 _ _ w988]
    tunnel: ["" w360 w427 w482 "" "" w683 w748 w826 w914 w1011] -> w27
    tunnel: "Search Parameters" -> [_ _ _ _ w538 w612 _ _ _ _ _]
    tunnel: w25 -> [_ _ w426 _ _ _ _ _ w815 w910 w992]
    tunnel: [_ _ _ _ _ _ _ _ w810 _ w1005] -> w24
    tunnel: w17 -> [_ _ _ _ _ _ w681 w747 _ _ _]
    tunnel: w6 -> [_ w359 _ _ _ _ _ _ _ _ _]
    tunnel: w4 -> [_ w356 _ _ _ _ _ _ _ _ _]
    tunnel: w2 -> [_ w340 _ _ _ _ _ _ _ _ _]
    frame "SELECT [Plant],[OrderNo]", Default {
      w151 = string[] ["Order No.", "Oper. No.", "Qty.", "NCR No.", "Customer No.", "Customer Name", "Project", "Sales Order", "Item No.", "Material", "Revision", "Material Description", "Serial No.", "UnitOfQty"]  # 2014-10-17 08:39 Item Details Label.Text
      w149 = string[] ["OrderNo", "OperationNo", "Qty", "NCRNo", "CustomerID", "Customer", "Project", "SalesOrderNo", "SalesOrderItemNo", "MaterialNo", "MaterialRev", "MaterialDesc", "SerialNos", "UnitOfQty"]  # 2014-10-17 08:39 [Config].[Mapping].[ColumnName]
      (unwired) string[] ["OrderNo", "OperationNo", "Qty", "NCRNo", "CustomerID", "Customer", "Project", "SalesOrderNo", "SalesOrderItemNo", "MaterialNo", "MaterialRev", "MaterialDesc", "SerialNos", "UnitOfQty"]  # 2014-10-17 08:39 [Config].[Mapping].[ColumnName]
      n55 = case shown="\"Interactive\", Default" w169 {
        tunnel: w165 -> [_ w285]
        tunnel: [w284 w285] -> w164
        frame "Interactive", Default {
          # "No Ref connected"
          n56 = control-ref of="Item Details"() -> (w284:refnum<vi>)
        }
        frame "subVI Mode" {
          # "External Cluster Ref Connected"
        }
      }
      n57 = Unbundle By Name(w173) -> ("Order No."=w172:string)
      n58 = Unbundle By Name(w171) -> ("PlantID"=w170:string)
      n59 = To Upper Case(1:w149) -> (0:w148:string[])
      n60 = call "DB - Replace DB.Schema.Table.vi"("DB.Schema.Table"=w150, "string in"="Use [<DB>]\n\nSELECT \n       [SourceTableName]\n      ,[SourceColumnName]\n      ,[IsMandatory]\n      ,[TargetColumnName]\nFROM [<Schema>].[<Table>]\nWHERE [TargetColumnName] \nIN (<Values>) \nAND [Inactive] = '0'\n") -> ("string out"=w161:string)  [unwired: 8 in, 1 out]
      n61 = call "DB - Array to Values.vi"("Array (0xFFFE autodetect)"=w154) -> ("<Values>"=w153:string)  [unwired: 10 in]
      n62 = Search and Replace String(replace all?=TRUE ("replace all? (F)"), input string=w161, search string="<Values>", replace string=w153) -> (result string=w168:string)  [unwired: 4 in, 3 out]
      n63 = call-poly <vilib>:"DB Tools Execute Query.vi"("error in (no error)"=w182, "SQL query"=w168, "connection reference"=w183) -> ("error out"=w160:errorcluster, "recordset reference"=w159:T20)  [unwired: 5 in]
      n64 = call-poly <vilib>:"DB Tools Fetch Recordset Data.vi"("error in (no error)"=w160, "recordset reference"=w159) -> ("error out"=w155:errorcluster, "recordset data"=w158:variant[][], "recordset reference out"=w156:T20)  [unwired: 3 in]
      n65 = xnode "Database Variant To Data"("database variant"=w158, "type"=string[][] []) -> ("data"=w152:string[][])  [unwired: 1 in, 1 out]
      n66 = call-poly <vilib>:"DB Tools Free Object.vi"("error in (no error)"=w155, "recordset reference"=w156) -> ("error out"=w177:errorcluster, "connection reference"=w178:T14)  [unwired: 8 in]
      n67 = global read "Global SRTRS.vi" "Logon Extra"() -> (w143:T21)
      n68 = Unbundle By Name(w143) -> ("IsUnicode"=w142:bool)
      n69 = call "DB - Replace DB.Schema.Table.vi"("DB.Schema.Table"=w150, "string in"="\nSELECT TOP 1 [<C>]\n  FROM [<DB>].[MasterData].[<T>]\nWHERE\n[PlantID] = '<A>' and [OrderNo] = '<B>'") -> ("string out"=w179:string)  [unwired: 8 in, 1 out]
      n70 = for {
        tunnel: w152 -> [w317] mode=indexing
        tunnel: w179 -> [w289]
        tunnel: w170 -> [w309]
        tunnel: w172 -> [w298]
        tunnel: w178 -> [w307]
        tunnel: w177 -> [w306]
        tunnel: [w305] -> w166 mode=indexing
        tunnel: [w304] -> w176
        tunnel: [w303] -> w175
        tunnel: [w302] -> w174 mode=indexing
        tunnel: [w295] -> w145 mode=indexing
        tunnel: [w291] -> w147 mode=indexing
        tunnel: w142 -> [w292]
        tunnel: [w286] -> w141 mode=indexing
        w288 = "<C>"  # Column
        w287 = string[] ["Customer", "Project", "MaterialDesc (NA)", "Notes (NA)"]  # 2014-12-03 15:18 [ColumnName] With Unicode
        w296 = 3  # [TargetColumnName]
        w299 = 2  # [IsMandatory]
        w300 = 1  # [SourceColumnName]
        w301 = 0  # [SourceTableName]
        w308 = "<B>"  # OrderNo
        w310 = "<A>"  # Plant
        n71 = Empty String/Path?(string/path=w298) -> (empty?=w297:bool)
        n72 = Index Array(array=w317, index #1=w301, index #2=w300, index #3=w299, index #4=w296) -> (element #1=w316:string, element #2=w314:string, element #3=w295:string, element #4=w291:string)
        n73 = Search 1D Array(1D array=w287, element=w291) -> (index of element=w294:i32)  [unwired: 1 in]
        n74 = Greater Or Equal To 0?(x=w294) -> (x >= 0?=w293:bool)
        n75 = And(x=w293, y=w292) -> (x .and. y?=w286:bool)
        n76 = case shown="True" w286 {
          tunnel: [w319 w322] -> w290
          tunnel: w289 -> [w319 w321]
          frame False {
          }
          frame True {
            w320 = "[<C>]"  # Column
            w323 = "CAST([<C>] AS varbinary(max))"  # Column (Unicode)
            n77 = Search and Replace String(input string=w321, search string=w320, replace string=w323) -> (result string=w322:string)  [unwired: 5 in, 3 out]
          }
        }
        n78 = Search and Replace String(input string=w290, search string="<T>", replace string=w316) -> (result string=w315:string)  [unwired: 5 in, 3 out]
        n79 = Search and Replace String(input string=w315, search string=w288, replace string=w314) -> (result string=w311:string)  [unwired: 5 in, 3 out]
        n80 = Search and Replace String(input string=w311, search string=w310, replace string=w309) -> (result string=w313:string, error out=w312:errorcluster)  [unwired: 5 in, 2 out]
        n81 = Search and Replace String(input string=w313, search string=w308, replace string=w298, error in=w312) -> (result string=w302:string)  [unwired: 4 in, 3 out]
        n82 = case shown="False" w297 {
          tunnel: w307 -> [w334 w337]
          tunnel: w306 -> [w333 w336]
          tunnel: [w328 ""] -> w305
          tunnel: [w327 w336] -> w304
          tunnel: [w326 w337] -> w303
          tunnel: w302 -> [w325 _]
          frame False {
            # "OrderNo NOT Blank"
            n83 = call-poly <vilib>:"DB Tools Execute Query.vi"("error in (no error)"=w333, "SQL query"=w325, "connection reference"=w334) -> ("error out"=w332:errorcluster, "recordset reference"=w331:T20)  [unwired: 5 in]
            n84 = call-poly <vilib>:"DB Tools Fetch Element Data.vi"("error in (no error)"=w332, "column index"=0, "recordset reference"=w331) -> ("error out"=w329:errorcluster, "data"=w328:string, "recordset reference out"=w330:T20)  [unwired: 4 in]
            n85 = call-poly <vilib>:"DB Tools Free Object.vi"("error in (no error)"=w329, "recordset reference"=w330) -> ("error out"=w327:errorcluster, "connection reference"=w326:T14)  [unwired: 8 in]
          }
          frame True {
            # "OrderNo Blank"
          }
        }
      }
      n86 = To Upper Case(1:w147) -> (0:w146:string[])
      n87 = for {
        tunnel: w146 -> [w234]
        tunnel: w148 -> [w233] mode=indexing
        tunnel: w166 -> [w238]
        tunnel: w164 -> [w241]
        tunnel: w151 -> [w237] mode=indexing
        tunnel: [w235] -> w140
        tunnel: w145 -> [w232]
        tunnel: [w231] -> w144 mode=indexing
        tunnel: w141 -> [w229]
        n88 = Search 1D Array(1D array=w234, element=w233) -> (index of element=w230:i32)  [unwired: 1 in]
        n89 = Index Array "Match [TargetColumnName]\n to Cluster Label"(array=w238, index=w230) -> (element=w239:string)
        n90 = Index Array "Match [TargetColumnName]\n to Cluster Label"(array=w229, index=w230) -> (element=w228:bool)
        n91 = Index Array "Match [TargetColumnName]\n to Cluster Label"(array=w232, index=w230) -> (element=w231:string)
        n92 = property class="Clust (strict)"(reference=w241) -> (error out=w236:errorcluster, "Controls[]"=w240:refnum<vi>[])  [unwired: 1 in, 1 out]
        n93 = for {
          tunnel: w240 -> [w254] mode=indexing
          tunnel: w239 -> [w252]
          tunnel: w237 -> [w251]
          tunnel: w236 -> [w246]
          tunnel: [w244] -> w235
          tunnel: w228 -> [w242]
          n94 = property class="Ctl"(reference=w254, error in=w246) -> (reference out=w253:refnum<vi>, error out=w245:errorcluster, "Label.Text"=w243:string)
          n95 = Not Equal?(x=w243, y="Order No.") -> (x != y?=w248:bool)
          n96 = Equal?(x=w243, y=w251) -> (x = y?=w249:bool)
          n97 = And(x=w249, y=w248) -> (x .and. y?=w247:bool)
          n98 = case shown="True" w247 {
            tunnel: w253 -> [_ w262]
            tunnel: w252 -> [_ w259]
            tunnel: w245 -> [_ w258]
            tunnel: [_ w256] -> w244
            tunnel: w242 -> [_ w255]
            frame False {
            }
            frame True {
              n99 = property class="Ctl"(reference=w262, error in=w258) -> (reference out=w260:refnum<vi>, error out=w257:errorcluster, "ClassName"=w261:string)
              n100 = case shown="\"String\", Default" w261 {
                tunnel: w260 -> [w270 w283]
                tunnel: w259 -> [w264 w280]
                tunnel: w257 -> [w268 w278]
                tunnel: [w267 w276] -> w256
                tunnel: w255 -> [w265 _]
                frame "String", Default {
                  w269 = refnum<vi> refnum  # String
                  n101 = To More Specific Class(target class=w269, reference=w270, error in=w268) -> (specific class reference=w266:refnum<vi>, error out=w263:errorcluster)
                  n102 = call "Tool_Unicode Update String.vi"("Interpret as Unicode (T)"=w265, "error in (no error)"=w263, "String Value"=w264, "String Control Reference"=w266) -> ()  [unwired: 4 in, 2 out]
                  n103 = disable-structure shown="Enabled" {
                    disable-tunnel: [w274 w275] -> w267
                    disable-tunnel: w266 -> [w273 _]
                    disable-tunnel: w264 -> [w272 _]
                    disable-tunnel: w263 -> [w271 w275]
                    frame Disabled {
                      n104 = property class="Str"(reference=w273, error in=w271, "Value"=w272) -> (error out=w274:errorcluster)  [unwired: 1 out]
                    }
                    frame Enabled {
                    }
                  }
                }
                frame "Digital" {
                  w282 = refnum<vi> refnum  # Digital
                  n105 = To More Specific Class(target class=w282, reference=w283, error in=w278) -> (specific class reference=w281:refnum<vi>, error out=w277:errorcluster)
                  n106 = Decimal String To Number(string=w280) -> (number=w279:i32)  [unwired: 2 in, 1 out]
                  n107 = property class="DigNum"(reference=w281, error in=w277, "Value"=w279) -> (error out=w276:errorcluster)  [unwired: 1 out]
                }
              }
            }
          }
        }
      }
      "[IsMandatory] Ordered" <- w144
      "Ref error out" <- w140
    }
    frame "INSERT [Setup].[Header]" {
      (unwired) "USE [<DB>]\n\nUPDATE [<Schema>].[<Table>]\n   SET <Values>\nWHERE [PlantId] = '<A>' AND\n[SystemId] = '<B>' AND\n[Inactive] = '0' \n\n"
      w342 = T22[] [enum."[PlantID]", enum."[SystemID]", enum."[ProcedureNo]", enum."[ProcedureRev]", enum."[WPSNo]", enum."[WPSRev]", enum."[HoldTemperature]", enum."[UnitOfTemperature]", enum."[HoldTime]", enum."[AdditionalProcs]", enum."[OutputSetId]", enum."[Equipment1ID]", enum."[Equipment2ID]", enum."[Equipment3ID]", enum."[Equipment4ID]", enum."[Equipment5ID]", enum."[Equipment6ID]", enum."[Equipment7ID]", enum."[Equipment8ID]", enum."[Equipment9ID]", enum."[Equipment10ID]", enum."[PermittedTempDiff]", enum."[PermittedTimeDiff]", enum."[Notes]", enum."[CreatedBy]", enum."[CreatedOn]", enum."[LastSavedBy]", enum."[LastSavedOn]"] items=["[TransactionNo]", "[PlantID]", "[SystemID]", "[ProcedureNo]", "[ProcedureRev]", "[WPSNo]", "[WPSRev]", "[HoldTemperature]", "[UnitOfTemperature]", "[HoldTime]", "[AdditionalProcs]", "[OutputSetId]", "[Equipment1ID]", "[Equipment2ID]", "[Equipment3ID]", "[Equipment4ID]", "[Equipment5ID]", "[Equipment6ID]", "[Equipment7ID]", "[Equipment8ID]", "[Equipment9ID]", "[Equipment10ID]", "[PermittedTempDiff]", "[PermittedTimeDiff]", "[Notes]", "[CreatedBy]", "[CreatedOn]", "[LastSavedBy]", "[LastSavedOn]"]
      w352 = 5 ("length (rest)")
      w358 = 5  # [EquipmentId]
      (unwired) string[] ["Name", "Model", "Serial No.", "Last Cal. Date", "Next Cal. Due Date", "[EquipmentId]"]  # 2014-09-29 09:49 Column Header Strings[]
      n108 = Empty String/Path?(string/path=w362) -> (empty?=w366:bool)
      n109 = case shown="True" w366 {
        tunnel: w365 -> [_ w413]
        tunnel: w364 -> [w403 w412]
        tunnel: [w403 w411] -> w363
        tunnel: [w402 w410] -> w360
        tunnel: w362 -> [w402 _]
        frame False {
          # "Existing [TransactionNo]"
        }
        frame True {
          w414 = "USE <DB>\n\nDECLARE @value as int\n\nEXEC GetNewTransactionNo  @transactionNo = @value OUTPUT, @reseedNo = <R>"  # Calling Stored Procedure GetNewTransactionNo
          # "Blank [TransactionNo]"
          n110 = global read "Global SRTRS.vi" "Transaction Start Number"() -> (w404:string)
          n111 = call "DB - Replace DB.Schema.Table.vi"("DB.Schema.Table"=w413, "string in"=w414) -> ("error out"=w406:errorcluster, "string out"=w409:string)  [unwired: 8 in]
          n112 = Search and Replace String(input string=w409, search string="<R>", replace string=w404, error in=w406) -> (result string=w408:string, error out=w405:errorcluster)  [unwired: 4 in, 2 out]
          n113 = call-poly <vilib>:"DB Tools Execute Query.vi"("error in (no error)"=w405, "SQL query"=w408, "connection reference"=w412) -> ("error out"=w417:errorcluster, "recordset reference"=w419:T20)  [unwired: 5 in]
          n114 = call-poly <vilib>:"DB Tools Fetch Element Data.vi"("error in (no error)"=w417, "column index"=0, "recordset reference"=w419) -> ("error out"=w416:errorcluster, "data"=w410:string, "recordset reference out"=w418:T20)  [unwired: 4 in]
          n115 = call-poly <vilib>:"DB Tools Free Object.vi"("error in (no error)"=w416, "recordset reference"=w418) -> ("connection reference"=w411:T14)  [unwired: 8 in, 1 out]
        }
      }
      n116 = disable-structure shown="Disabled" {
        frame Disabled {
          (unwired) "SELECT SCOPE_IDENTITY()" ("SQL query")
          n117 = call-poly <vilib>:"DB Tools Fetch Element Data.vi"() -> ()  [unwired: 7 in, 3 out]
          n118 = call-poly <vilib>:"DB Tools Fetch Recordset Data.vi"() -> ()  [unwired: 5 in, 3 out]
        }
        frame Enabled {
        }
      }
      n119 = Unbundle By Name(w356) -> ("Variant Allowed (Hold Temp)"=w355:dbl, "Variant Allowed (Hold Time)"=w349:dbl)
      n120 = Index Array(array=w359, index (col)=w358) -> (element=w357:string[])  [unwired: 1 in]
      n121 = Unbundle By Name(w396) -> ("PlantID"=w373:string, "SystemID"=w372:string, "UserID"=w348:string)  [unwired: 2 out]
      n122 = Unbundle By Name(w395) -> ("WPS/Ref"=w394:T1, "Rev"=w393:T1, "Hold Temperature"=w390:string, "WPS Details Temperature Units"=w389:string, "Hold Time (HH:MM)"=w388:string)
      n123 = Number To Decimal String(number=w349) -> (decimal integer string=w353:string)  [unwired: 1 in]
      n124 = Number To Decimal String(number=w355) -> (decimal integer string=w354:string)  [unwired: 1 in]
      n125 = Unbundle By Name(w340) -> ("Output Set"=w339:T1)
      n126 = global read "Global SRTRS.vi" "Date Time Format"() -> (w346:string)
      n127 = Array To Spreadsheet String(delimiter (Tab)=",", array=w387, 3:"" ("format string")) -> (spreadsheet string=w384:string)
      n128 = String Subset(string=w354, length (rest)=w352) -> (substring=w351:string)  [unwired: 1 in]
      n129 = String Subset(string=w353, length (rest)=w352) -> (substring=w350:string)  [unwired: 1 in]
      n130 = Initialize Array("NULL", 10 ("dimension size")) -> (w381:string[])
      n131 = Format Date/Time String(time format string (%c)=w346) -> (date/time string=w347:string)  [unwired: 2 in]
      n132 = Replace Array Subset(array=w381, new element=w357) -> (w379:string[])  [unwired: 1 in]
      n133 = Build Array(w351, w350, w377, w348, w347, w348, w347) -> (w378:string[])
      n134 = Build Array(w373, w372, w394, w393, w392, w391, w390, w389, w388, w384, w339) -> (w380:T1[])
      n135 = Build Array (concatenate)(w380, w379, w378) -> (w343:T1[])
      n136 = call "DB - Replace DB.Schema.Table.vi"("DB.Schema.Table"=w365, "string in"="USE [<DB>]\n\nUPDATE [<Schema>].[<Table>]\n   SET <Values>\nWHERE [TransactionNo] = '<A>' \nAND\n[Inactive] = '0' \n\n") -> ("error out"=w398:errorcluster, "string out"=w399:string)  [unwired: 8 in]
      n137 = for {
        tunnel: w342 -> [w401] mode=indexing
        tunnel: [w400] -> w341 mode=indexing
        n138 = Format Into String(w401) -> (resulting string=w400:string)  [unwired: 3 in, 1 out]
      }
      n139 = call "DB - Update [Table] Set [ColNames] equ Data.vi"("<Data> (0xFFFE autodetect)"=w343, "[ColumnNames]"=w341) -> ("<Values>"=w345:string)  [unwired: 9 in]
      n140 = Search and Replace String(input string=w399, search string="<Values>", replace string=w345, error in=w398) -> (result string=w371:string)  [unwired: 4 in, 3 out]
      n141 = Search and Replace String(replace all?=TRUE ("replace all? (F)"), input string=w371, search string="<A>", replace string=w360) -> (result string=w361:string)  [unwired: 4 in, 3 out]
      n142 = call-poly <vilib>:"DB Tools Execute Query.vi"("error in (no error)"=w376, "SQL query"=w361, "connection reference"=w363) -> ("error out"=w374:errorcluster, "recordset reference"=w375:T20)  [unwired: 5 in]
      n143 = call-poly <vilib>:"DB Tools Free Object.vi"("error in (no error)"=w374, "recordset reference"=w375) -> ("error out"=w367:errorcluster, "connection reference"=w368:T14)  [unwired: 8 in]
      n144 = Build Array(w361) -> (w338:string[])
    }
    frame "INSERT [Setup].[Item]" {
      w420 = "USE [<DB>]\n\nIF EXISTS(SELECT 1 from [<Schema>].[<Table>]\nWHERE [TransactionNo] = '<A>'  <CONDITION>)\n\nBEGIN\nDELETE FROM [<Schema>].[<Table>]\nWHERE  [TransactionNo] = '<A>'  <CONDITION>\nEND\n\nINSERT INTO [<Schema>].[<Table>]\n           ([TransactionNo]\n              <B>\n            ,[ItemNo]\n           ,[OrderNo]\n           ,[OperationNo]\n           ,[Qty]\n           ,[UnitOfQty]\n           ,[NCRIndicator]\n           ,[NCRNo]\n           ,[CustomerID]\n           ,[Customer]\n           ,[Project]\n           ,[SalesOrderNo]\n           ,[SalesOrderItemNo]\n           ,[MaterialNo]\n           ,[MaterialDesc]\n           ,[MaterialRev]\n           ,[SerialNos]\n           ,[Notes]\n           ,[TC01]  ,[TC02]  ,[TC03] ,[TC04] ,[TC05] ,[TC06] \n           ,[TC01Plot] ,[TC02Plot] ,[TC03Plot] ,[TC04Plot] ,[TC05Plot] ,[TC06Plot] \n           )\nVALUES (<Values>)\n\n"  # 30 Columns
      n145 = Equal?(x="", y=w426) -> (x = y?=w424:bool)
      n146 = case shown="False" w424 {
        tunnel: w427 -> [w467 w470]
        tunnel: w426 -> [w464 _]
        tunnel: [w466 w469] -> w425
        tunnel: [w462 w468] -> w423
        tunnel: [",[TransactionRunNo]" w468] -> w422
        frame False {
          # "[TransactionRunNo] Exists"
          n147 = Build Array(w467, w464) -> (w466:string[])
          n148 = Concatenate Strings("AND [TransactionRunNo] = '", w464, "'" ("string")) -> (w462:string)
        }
        frame True {
          w468 = ""
          # "BLANK"
          n149 = Build Array(w470) -> (w469:string[])
        }
      }
      n150 = call "DB - Sort Item Names To DB.vi"("ItemNames"=w452) -> ("DB Query Array"=w451:string[][])  [unwired: 9 in, 1 out]
      n151 = for {
        tunnel: w425 -> [w477]
        tunnel: w451 -> [w476] mode=indexing
        shift-right: [w479] -> w450
        shift-left: "" -> [w473]
        tunnel: [w478] -> _
        i -> [w478]
        n152 = Greater Than 0?(x=w478) -> (x > 0?=w481:bool)
        n153 = Build Array (concatenate)(w477, w476) -> (w475:string[])
        n154 = Select(t="), (", s=w481, f="") -> (s? t:f=w472:string)
        n155 = call "DB - Array to Values.vi"("Array (0xFFFE autodetect)"=w475) -> ("<Values>"=w474:string)  [unwired: 10 in]
        n156 = Concatenate Strings(w473, w472, w474) -> (w479:string)
      }
      n157 = call "DB - Replace DB.Schema.Table.vi"("DB.Schema.Table"=w459, "string in"=w420) -> ("string out"=w429:string)  [unwired: 8 in, 1 out]
      n158 = disable-structure shown="Disabled" {
        frame Disabled {
          (unwired) "CONVERT(varbinary(max),'<D>',1)"  # Column (Unicode)
          (unwired) string[] ["Customer", "Project", "MaterialDesc", "Notes"]  # 2014-12-03 15:18 [ColumnName] With Unicode
          n159 = global read "Global SRTRS.vi" "Logon Extra"() -> (w460:T21)
          n160 = call "String - Unicode String to Hex String.vi"() -> ()  [unwired: 11 in, 1 out]
          n161 = Unbundle By Name(w460) -> ()  [unwired: 1 out]
        }
        frame Enabled {
        }
      }
      n162 = Search and Replace String(replace all?=TRUE ("replace all? (F)"), input string=w429, search string="<A>", replace string=w427) -> (result string=w428:string)  [unwired: 4 in, 3 out]
      n163 = Search and Replace String(replace all?=TRUE ("replace all? (F)"), input string=w428, search string="<CONDITION>", replace string=w423) -> (result string=w435:string)  [unwired: 4 in, 3 out]
      n164 = Search and Replace String(replace all?=TRUE ("replace all? (F)"), input string=w435, search string="<B>", replace string=w422) -> (result string=w432:string)  [unwired: 4 in, 3 out]
      n165 = Search and Replace String(input string=w432, search string="<Values>", replace string=w450) -> (result string=w431:string)  [unwired: 5 in, 3 out]
      n166 = Search and Replace String(replace all?=TRUE ("replace all? (F)"), input string=w431, search string="'TRUE'", replace string="1" ("replace string (\"\")")) -> (result string=w447:string)  [unwired: 4 in, 3 out]
      n167 = Search and Replace String(replace all?=TRUE ("replace all? (F)"), input string=w447, search string="'FALSE'", replace string="0" ("replace string (\"\")")) -> (result string=w430:string)  [unwired: 4 in, 3 out]
      n168 = call-poly <vilib>:"DB Tools Execute Query.vi"("error in (no error)"=w456, "SQL query"=w430, "connection reference"=w457) -> ("error out"=w439:errorcluster, "recordset reference"=w440:T20)  [unwired: 5 in]
      n169 = call-poly <vilib>:"DB Tools Free Object.vi"("error in (no error)"=w439, "recordset reference"=w440) -> ("error out"=w454:errorcluster, "connection reference"=w455:T14)  [unwired: 8 in]
      n170 = Build Array(w430) -> (w421:string[])
    }
    frame "INSERT [Setup].[ProcedureItem]" {
      (unwired) ""
      n171 = Unbundle By Name(w484) -> ("WPS Details Temperature Units"=w483:string)
      n172 = Array Size(array=w485) -> (size(s)=w493:i32[])
      n173 = Index Array(array=w493) -> (element=w494:i32)  [unwired: 1 in]
      n174 = Decrement "Exclude Last Row (which is blank)"(x=w494) -> (x-1=w495:i32)
      n175 = for {
        N: w495 -> [_]
        tunnel: w485 -> [w527] mode=indexing
        shift-right: [w530] -> w488
        shift-left: "" -> [w531]
        tunnel: w483 -> [w526]
        w522 = "<A>"  # [TransactionNo]
        w524 = "0"  # Inactive
        w528 = 2  # unitRampRate
        n176 = Insert Into Array(array=w527, index=w528, new element=w526) -> (w525:string[])
        n177 = Build Array (concatenate)(w522, w525, w524) -> (w523:string[])
        n178 = Array To Spreadsheet String(delimiter (Tab)="','", array=w523, 3:"" ("format string")) -> (spreadsheet string=w529:string)
        n179 = Concatenate Strings(w531, ",('" ("string"), w529, "')" ("string")) -> (w530:string)
      }
      n180 = String Subset "Skip 1st ,"(string=w488, offset (0)=1) -> (substring=w490:string)  [unwired: 1 in]
      n181 = call "DB - Replace DB.Schema.Table.vi"("DB.Schema.Table"=w511, "string in"="USE [<DB>]\n\nIF EXISTS(SELECT 1 from [<Schema>].[<Table>] \nwhere [TransactionNo] = '<A>' )\nBEGIN\nDELETE FROM [<Schema>].[<Table>] \n      WHERE [TransactionNo] = '<A>'\nEND\n\nINSERT INTO [<Schema>].[<Table>] \n           ([TransactionNo]\n           ,[SequenceNo]\n           ,[rampRate]\n           ,[unitRampRate]\n           ,[targetTemperature]\n           ,[holdTimeDuration]\n           ,[Inactive]\n           )\n     VALUES\n           (<Values>)") -> ("error out"=w509:errorcluster, "string out"=w510:string)  [unwired: 8 in]
      n182 = Search and Replace String(replace all?=TRUE ("replace all? (F)"), input string=w490, search string="\r\n") -> (result string=w486:string)  [unwired: 5 in, 3 out]
      n183 = Search and Replace String(input string=w510, search string="(<Values>)", replace string=w486, error in=w509) -> (result string=w503:string)  [unwired: 4 in, 3 out]
      n184 = Search and Replace String(replace all?=TRUE ("replace all? (F)"), input string=w503, search string="<A>", replace string=w482) -> (result string=w500:string)  [unwired: 4 in, 3 out]
      n185 = disable-structure shown="Disabled" {
        disable-tunnel: w500 -> [w520 w521]
        disable-tunnel: [w512 w521] -> w496
        frame Disabled {
          n186 = Search and Replace String(replace all?=TRUE ("replace all? (F)"), input string=w520, search string="'TRUE'", replace string="1" ("replace string (\"\")")) -> (result string=w519:string)  [unwired: 4 in, 3 out]
          n187 = Search and Replace String(replace all?=TRUE ("replace all? (F)"), input string=w519, search string="'FALSE'", replace string="0" ("replace string (\"\")")) -> (result string=w512:string)  [unwired: 4 in, 3 out]
        }
        frame Enabled {
        }
      }
      n188 = call-poly <vilib>:"DB Tools Execute Query.vi"("error in (no error)"=w506, "SQL query"=w496, "connection reference"=w507) -> ("error out"=w498:errorcluster, "recordset reference"=w499:T20)  [unwired: 5 in]
      n189 = call-poly <vilib>:"DB Tools Free Object.vi"("error in (no error)"=w498, "recordset reference"=w499) -> ("error out"=w504:errorcluster, "connection reference"=w505:T14)  [unwired: 8 in]
    }
    frame "SELECT [TransactionNo]" {
      n190 = String Length(string=w538) -> (length=w544:i32)
      n191 = Equal To 0?(x=w544) -> (x = 0?=w545:bool)
      n192 = Select(t="%", s=w545, f=w538) -> (s? t:f=w542:string)
      n193 = Search and Replace String(replace all?=TRUE ("replace all? (F)"), input string=w542, search string=";", replace string="") -> (result string=w539:string)  [unwired: 4 in, 3 out]
      n194 = call "DB - Replace DB.Schema.Table.vi"("DB.Schema.Table"=w558, "string in"="USE [<DB>]\n\nSELECT TOP 100  [TransactionNo]\n     \nFROM [<Schema>].[<Table>]\n\nWHERE [Inactive] = '0' AND\n[TransactionNo] LIKE '<CONDITION>'\n\nORDER BY [TransactionNo] DESC") -> ("error out"=w547:errorcluster, "string out"=w550:string)  [unwired: 8 in]
      n195 = Search and Replace String(input string=w550, search string="<CONDITION>", replace string=w539, error in=w547) -> (result string=w548:string, error out=w546:errorcluster)  [unwired: 4 in, 2 out]
      n196 = call-poly <vilib>:"DB Tools Execute Query.vi"("error in (no error)"=w546, "SQL query"=w548, "connection reference"=w556) -> ("error out"=w565:errorcluster, "recordset reference"=w564:T20)  [unwired: 5 in]
      n197 = call-poly <vilib>:"DB Tools Fetch Recordset Data.vi"("error in (no error)"=w565, "recordset reference"=w564) -> ("error out"=w559:errorcluster, "recordset data"=w563:variant[][], "recordset reference out"=w560:T20)  [unwired: 3 in]
      n198 = xnode "Database Variant To Data"("database variant"=w563, "type"=string[][] []) -> ("data"=w561:string[][])  [unwired: 1 in, 1 out]
      n199 = call-poly <vilib>:"DB Tools Free Object.vi"("error in (no error)"=w559, "recordset reference"=w560) -> ("error out"=w554:errorcluster, "connection reference"=w555:T14)  [unwired: 8 in]
      n200 = Index Array(array=w561, index (col)=0 ("index (row)")) -> (element=w553:string[])  [unwired: 1 in]
      n201 = Build Array(w548) -> (w536:string[])
    }
    frame "SELECT [OrderNo]" {
      (unwired) "USE [<DB>]\n\nSELECT TOP 100  [TransactionNo]\n     \nFROM [<Schema>].[<Table>]\n\nWHERE [Inactive] = '0' AND\n[TransactionNo] LIKE '<CONDITION>'\n\nORDER BY [TransactionNo] DESC"
      n202 = String Length(string=w612) -> (length=w620:i32)
      n203 = Equal To 0?(x=w620) -> (x = 0?=w621:bool)
      n204 = Select(t="%", s=w621, f=w612) -> (s? t:f=w618:string)
      n205 = Search and Replace String(replace all?=TRUE ("replace all? (F)"), input string=w618, search string=";", replace string="") -> (result string=w611:string)  [unwired: 4 in, 3 out]
      n206 = call "DB - Replace DB.Schema.Table.vi"("DB.Schema.Table"=w629, "string in"="USE [<DB>]\n\nSELECT TOP 100 [OrderNo]\n     \nFROM [<Schema>].[<Table>]\n\nWHERE [Inactive] = '0' AND\n[OrderNo] LIKE '<CONDITION>'\n \nGROUP BY [OrderNo]\nORDER BY [OrderNo] DESC") -> ("string out"=w615:string)  [unwired: 8 in, 1 out]
      n207 = Search and Replace String(input string=w615, search string="<CONDITION>", replace string=w611) -> (result string=w614:string)  [unwired: 5 in, 3 out]
      n208 = call-poly <vilib>:"DB Tools Execute Query.vi"("SQL query"=w614, "connection reference"=w627) -> ("error out"=w636:errorcluster, "recordset reference"=w635:T20)  [unwired: 6 in]
      n209 = call-poly <vilib>:"DB Tools Fetch Recordset Data.vi"("error in (no error)"=w636, "recordset reference"=w635) -> ("error out"=w630:errorcluster, "recordset data"=w634:variant[][], "recordset reference out"=w631:T20)  [unwired: 3 in]
      n210 = xnode "Database Variant To Data"("database variant"=w634, "type"=string[][] []) -> ("data"=w632:string[][])  [unwired: 1 in, 1 out]
      n211 = call-poly <vilib>:"DB Tools Free Object.vi"("error in (no error)"=w630, "recordset reference"=w631) -> ("error out"=w625:errorcluster, "connection reference"=w626:T14)  [unwired: 8 in]
      n212 = Index Array(array=w632, index (col)=0 ("index (row)")) -> (element=w624:string[])  [unwired: 1 in]
    }
    frame "SELECT [TransactionNo], others" {
      n213 = call "DB - Replace DB.Schema.Table.vi"("DB.Schema.Table 4"=w681, "DB.Schema.Table 3"=w684, "DB.Schema.Table 2"=w688, "DB.Schema.Table"=w694, "string in"="USE [<DB>]\n\nSELECT  f.[CreatedOn], f.[TransactionNo], NULL AS [TransactionRunNo], g.[OrderNo] AS [OrderNo]\nFROM [<Schema>].[<Table>] as f\nRIGHT JOIN [<Schema2>].[<Table2>] as g \nON f.[TransactionNo] = g.[TransactionNo]\nWHERE  f.[Inactive] = '0' AND g.[Inactive] = '0' AND  f.[TransactionNo] = '<A>'\n\nUNION\n\nSELECT  h.[LastSavedOn] AS [CreatedOn], h.[TransactionNo], h.[TransactionRunNo], i.[OrderNo]\nFROM [<Schema3>].[<Table3>] as h\nRIGHT JOIN [<Schema4>].[<Table4>] as i\nON h.[TransactionNo] = i.[TransactionNo] AND\nh.[TransactionRunNo] = i.[TransactionRunNo]\n\nWHERE h.[Inactive] = '0' AND i.[Inactive] = '0' AND h.[TransactionNo] = '<A>' \n\nORDER BY [CreatedOn] DESC\n\n") -> ("string out"=w689:string)  [unwired: 5 in, 1 out]
      n214 = Search and Replace String(replace all?=TRUE, input string=w689, search string="<A>", replace string=w683) -> (result string=w685:string)  [unwired: 4 in, 3 out]
      n215 = call-poly <vilib>:"DB Tools Execute Query.vi"("SQL query"=w685, "connection reference"=w692) -> ("error out"=w700:errorcluster, "recordset reference"=w699:T20)  [unwired: 6 in]
      n216 = call-poly <vilib>:"DB Tools Fetch Recordset Data.vi"("error in (no error)"=w700, "recordset reference"=w699) -> ("error out"=w695:errorcluster, "recordset data"=w698:variant[][], "recordset reference out"=w696:T20)  [unwired: 3 in]
      n217 = xnode "Database Variant To Data"("database variant"=w698, "type"=string[][] []) -> ("data"=w686:string[][])  [unwired: 1 in, 1 out]
      n218 = call-poly <vilib>:"DB Tools Free Object.vi"("error in (no error)"=w695, "recordset reference"=w696) -> ("error out"=w690:errorcluster, "connection reference"=w691:T14)  [unwired: 8 in]
    }
    frame "SELECT [OrderNo], others" {
      w748 = ""  # No [TransactionNo] when Choosing [OrderNo]s
      (unwired) "USE [<DB>]\n\nSELECT  h.[CreatedOn],  h.[TransactionNo], k.[TransactionRunNo], i.[OrderNo]\n     \nFROM [<Schema>].[<Table>] as h\nRIGHT JOIN [<Schema2>].[<Table2>] as i\nON h.[TransactionNo] = i.[TransactionNo]\nRIGHT JOIN [<Schema3>].[<Table3>] as k\nON h.[TransactionNo] = k.[TransactionNo]\n\nWHERE h.[Inactive] = '0' AND i.[Inactive] = '0' AND \ni.[OrderNo] = '<A>'\n\nORDER BY i.[OrderNo] DESC\n "
      n219 = call "DB - Replace DB.Schema.Table.vi"("DB.Schema.Table 4"=w747, "DB.Schema.Table 3"=w749, "DB.Schema.Table 2"=w754, "DB.Schema.Table"=w759, "string in"="USE [<DB>]\n\nSELECT  f.[CreatedOn], f.[TransactionNo], NULL AS [TransactionRunNo], g.[OrderNo] AS [OrderNo]\nFROM [<Schema>].[<Table>] as f\nRIGHT JOIN [<Schema2>].[<Table2>] as g \nON f.[TransactionNo] = g.[TransactionNo]\n\nWHERE f.[Inactive] = '0' AND g.[Inactive]='0' AND  g.[OrderNo] = '<A>'\n\nUNION\n\nSELECT  h.[LastSavedOn] AS [CreatedOn], h.[TransactionNo], h.[TransactionRunNo], i.[OrderNo]\nFROM [<Schema3>].[<Table3>] as h\nRIGHT JOIN [<Schema4>].[<Table4>] as i\nON h.[TransactionNo] = i.[TransactionNo] AND\nh.[TransactionRunNo] = i.[TransactionRunNo]\n\nWHERE h.[Inactive] = '0' AND i.[Inactive]='0' AND i.[OrderNo] = '<A>' \n\nORDER BY [CreatedOn] DESC\n\n") -> ("string out"=w755:string)  [unwired: 5 in, 1 out]
      n220 = Search and Replace String(replace all?=TRUE, input string=w755, search string="<A>", replace string=w750) -> (result string=w751:string)  [unwired: 4 in, 3 out]
      n221 = call-poly <vilib>:"DB Tools Execute Query.vi"("SQL query"=w751, "connection reference"=w758) -> ("error out"=w765:errorcluster, "recordset reference"=w764:T20)  [unwired: 6 in]
      n222 = call-poly <vilib>:"DB Tools Fetch Recordset Data.vi"("error in (no error)"=w765, "recordset reference"=w764) -> ("error out"=w760:errorcluster, "recordset data"=w763:variant[][], "recordset reference out"=w761:T20)  [unwired: 3 in]
      n223 = xnode "Database Variant To Data"("database variant"=w763, "type"=string[][] []) -> ("data"=w752:string[][])  [unwired: 1 in, 1 out]
      n224 = call-poly <vilib>:"DB Tools Free Object.vi"("error in (no error)"=w760, "recordset reference"=w761) -> ("error out"=w756:errorcluster, "connection reference"=w757:T14)  [unwired: 8 in]
    }
    frame "SELECT [Setup].[ProcedureItem]" {
      n225 = String Length(string=w815) -> (length=w825:i32)
      n226 = Greater Than 0?(x=w825) -> (x > 0?=w824:bool)
      n227 = Search and Replace String(input string="AND [TransactionRunNo] = '<B>'", search string="<B>", replace string=w815) -> (result string=w821:string)  [unwired: 5 in, 3 out]
      n228 = Select(t=w821, s=w824, f="") -> (s? t:f=w819:string)
      n229 = call "DB - Replace DB.Schema.Table.vi"("DB.Schema.Table"=w839, "string in"="USE [<DB>]\n\n\nSELECT \n       [SequenceNo]\n      ,[RampRate]\n      ,[TargetTemperature]\n      ,[HoldTimeDuration]\n     FROM [<Schema>].[<Table>]\n\nWHERE [TransactionNo] = '<A>'\n<CONDITION>\n\n") -> ("string out"=w832:string)  [unwired: 8 in, 1 out]
      n230 = Search and Replace String(input string=w832, search string="<A>", replace string=w826) -> (result string=w818:string)  [unwired: 5 in, 3 out]
      n231 = Initialize Array("", 4 ("dimension size")) -> (w828:string[])
      n232 = Search and Replace String(input string=w818, search string="<CONDITION>", replace string=w819) -> (result string=w817:string)  [unwired: 5 in, 3 out]
      n233 = call-poly <vilib>:"DB Tools Execute Query.vi"("SQL query"=w817, "connection reference"=w837) -> ("error out"=w845:errorcluster, "recordset reference"=w844:T20)  [unwired: 6 in]
      n234 = call-poly <vilib>:"DB Tools Fetch Recordset Data.vi"("error in (no error)"=w845, "recordset reference"=w844) -> ("error out"=w840:errorcluster, "recordset data"=w843:variant[][], "recordset reference out"=w841:T20)  [unwired: 3 in]
      n235 = xnode "Database Variant To Data"("database variant"=w843, "type"=string[][] []) -> ("data"=w812:string[][])  [unwired: 1 in, 1 out]
      n236 = call-poly <vilib>:"DB Tools Free Object.vi"("error in (no error)"=w840, "recordset reference"=w841) -> ("error out"=w835:errorcluster, "connection reference"=w836:T14)  [unwired: 8 in]
      n237 = Build Array (concatenate)(w812, w828) -> (w827:string[][])
      n238 = call "VI - Interactive or SubVI.vi"() -> ("Mode"=w834:T16)  [unwired: 5 in]
      n239 = property on="MCListBox FHS Setup" class="MCListbox (strict)"("ItemNames"=w827) -> ()  [unwired: 2 in, 2 out]
      n240 = case shown="\"subVI Mode\"" w834 {
        tunnel: w833 -> [_ w854]
        tunnel: w827 -> [_ w853]
        frame "Interactive", Default {
        }
        frame "subVI Mode" {
          n241 = property class="MCListbox (strict)"(reference=w854, "ItemNames"=w853) -> (error out=w852:errorcluster)  [unwired: 1 in, 1 out]
          n242 = local write "Refnums error out"(w852) -> ()
        }
      }
      n243 = Transpose 2D Array(2D array=w812) -> (transposed array=w814:string[][])
      n244 = for {
        tunnel: w814 -> [w851] mode=indexing
        shift-right: [w848] -> w811
        shift-left: "" -> [w850]
        n245 = Array To Spreadsheet String(delimiter (Tab)=",", array=w851, 3:"" ("format string")) -> (spreadsheet string=w849:string)
        n246 = Concatenate Strings(w850, w849) -> (w848:string)
      }
      n247 = Build Array(w811) -> (w810:string[])
    }
    frame "SELECT [EquipmentxId]" {
      n248 = call "DB - Replace DB.Schema.Table.vi"("DB.Schema.Table"=w921, "string in"="USE [<DB>]\n\nSELECT\n[PlantId],[SystemId], \n[Equipment1Id],[Equipment2Id],[Equipment3Id],[Equipment4Id],[Equipment5Id],\n[Equipment6Id],[Equipment7Id],[Equipment8Id],[Equipment9Id],[Equipment10Id]\n   \n     FROM [<Schema>].[<Table>]\n\nWHERE [TransactionNo] = '<A>' AND [TransactionRunNo] =  '<B>' AND [Inactive] = '0'\n\n") -> ("string out"=w916:string)  [unwired: 8 in, 1 out]
      n249 = Search and Replace String(input string=w916, search string="<A>", replace string=w914) -> (result string=w913:string)  [unwired: 5 in, 3 out]
      n250 = Search and Replace String(input string=w913, search string="<B>", replace string=w910) -> (result string=w912:string)  [unwired: 5 in, 3 out]
      n251 = call-poly <vilib>:"DB Tools Execute Query.vi"("SQL query"=w912, "connection reference"=w919) -> ("error out"=w927:errorcluster, "recordset reference"=w926:T20)  [unwired: 6 in]
      n252 = call-poly <vilib>:"DB Tools Fetch Recordset Data.vi"("error in (no error)"=w927, "recordset reference"=w926) -> ("error out"=w922:errorcluster, "recordset data"=w925:variant[][], "recordset reference out"=w923:T20)  [unwired: 3 in]
      n253 = xnode "Database Variant To Data"("database variant"=w925, "type"=string[][] []) -> ("data"=w909:string[][])  [unwired: 1 in, 1 out]
      n254 = call-poly <vilib>:"DB Tools Free Object.vi"("error in (no error)"=w922, "recordset reference"=w923) -> ("error out"=w917:errorcluster, "connection reference"=w918:T14)  [unwired: 8 in]
      n255 = Index Array(array=w909, index (row)=0) -> (element=w901:string[])  [unwired: 1 in]
      n256 = Array Subset(array=w901, index=2) -> (w899:string[])  [unwired: 1 in]
      n257 = Index Array(array=w901, index #1=0 ("index"), index #2=1 ("index")) -> (element #1=w904:string, element #2=w902:string)
      n258 = call "DB - Array to Values.vi"("Array (0xFFFE autodetect)"=w899) -> ("<Values>"=w908:string)  [unwired: 10 in]
      n259 = Build Array(w904, w902, w908) -> (w907:string[])
    }
    frame "SELECT h.[TransactionNo], i.[OrderNo]" {
      w1030 = 0  # row (from row0)
      (unwired) string[] ["No.", "Order No.", "Oper. No.", "Qty.", "UnitOfQty", "NCR Boolean", "NCR No.", "Customer No.", "Customer Name", "Project", "Sales Order", "Item No.", "Material", "Material Description", "Revision", "Serial No.", "Notes", "TC1", "TC2", "TC3", "TC4", "TC5", "TC6", "TC01Plot", "TC02Plot", "TC03Plot", "TC04Plot", "TC05Plot", "TC06Plot"]  # 2014-09-06 [Setup].[itemNo]
      (unwired) string[] ["No.", "Order No.", "Oper. No.", "Qty.", "NCR No.", "Customer Name", "Project", "Sales Order", "Item No.", "Material", "Material Description", "Revision", "Serial No.", "TC1", "TC2", "TC3", "TC4", "TC5", "TC6", "Notes", "User", "Customer No.", "NCR Boolean", "UnitOfQty", "TC01Plot", "TC02Plot", "TC03Plot", "TC04Plot", "TC05Plot", "TC06Plot"]  # 2014-09-06 MClistBox Col Hdr[]
      n260 = String Length(string=w992) -> (length=w1008:i32)
      n261 = Concatenate Strings("AND h.[TransactionRunNo] = '", w992, "'") -> (w990:string)
      n262 = Greater Than 0?(x=w1008) -> (x > 0?=w996:bool)
      n263 = Select(t=w990, s=w996, f="") -> (s? t:f=w1006:string)
      n264 = Select(t="AND h.[TransactionRunNo] = i.[TransactionRunNo]", s=w996, f="") -> (s? t:f=w995:string)
      n265 = Unbundle By Name(w1046) -> ("WPS Details"=w1045:refnum<vi>, "WPS (Extra)"=w1038:refnum<vi>, "Rev (Extra)"=w1036:refnum<vi>, "Additional WPS/Ref MCListBox"=w1024:refnum<vi>, "Part Details (MClistBox)"=w1027:refnum<vi>, "Result Output"=w986:refnum<vi>)  [unwired: 2 out]
      n266 = global read "Global SRTRS.vi" "Logon Extra"() -> (w975:T21)
      n267 = Unbundle By Name(w975) -> ("IsUnicode"=w972:bool)
      n268 = case shown="True" w972 {
        tunnel: "USE [<DB>]\n\nSELECT   \n             h.[TransactionNo]\n             ,h.[ProcedureNo]\n             ,h.[ProcedureRev]\n             ,h.[WPSNo]\n             ,h.[WPSRev]\n             ,h.[HoldTemperature]\n             ,h.[UnitOfTemperature]\n             ,h.[HoldTime]\n             ,h.[AdditionalProcs]\n             ,h.[OutputSetId]\n             ,h.[PermittedTempDiff]\n             ,h.[PermittedTimeDiff]\n             ,j.[Description]\n          ,i.[itemNo] \n          ,i.[OrderNo]\n          ,i.[OperationNo]\n          ,i.[Qty]\n          ,i.[UnitOfQty]\n          ,i.[NCRIndicator]\n          ,i.[NCRNo]\n          ,i.[CustomerID]\n          ,i.[Customer]\n          ,i.[Project]\n          ,i.[SalesOrderNo]\n          ,i.[SalesOrderItemNo]\n          ,i.[MaterialNo]\n          ,i.[MaterialDesc]\n          ,i.[MaterialRev]\n          ,i.[SerialNos]\n          ,i.[Notes]\n          ,i.[TC01]\n          ,i.[TC02]\n          ,i.[TC03]\n          ,i.[TC04]\n          ,i.[TC05]\n          ,i.[TC06]\n          ,i.[TC01Plot]\n          ,i.[TC02Plot]\n          ,i.[TC03Plot]\n          ,i.[TC04Plot]\n          ,i.[TC05Plot]\n          ,i.[TC06Plot]\n                 \nFROM [<Schema>].[<Table>] as h\n\nRIGHT JOIN [<Schema2>].[<Table2>] as i ON \nh.[TransactionNo] = i.[TransactionNo]\n<CONDITION1>\n\nLEFT JOIN [<Schema3>].[<Table3>] as j ON \nh.[OutputSetId] = j.[OutputSetId] AND\nh.[PlantId] = j.[PlantId]\n\nWHERE h.[Inactive] = '0' AND i.[Inactive] = '0' AND j.[Inactive] = '0'\nAND h.[TransactionNo] = '<A>' <CONDITION2>\n\nORDER BY i.[itemNo] " -> [w1061 w1063]
        tunnel: [w1061 w1062] -> w973
        frame False {
        }
        frame True {
          w1064 = string[] ["Customer", "Project", "MaterialDesc", "Notes"]  # 2014-12-03 15:18 [ColumnName] With Unicode
          n269 = for {
            tunnel: w1064 -> [w1072] mode=indexing
            shift-right: [w1065] -> w1062
            shift-left: w1063 -> [w1070]
            w1069 = "CAST([<C>] AS varbinary(max))"  # Column (Unicode)
            n270 = Concatenate Strings("i.[" ("string"), w1072, "]" ("string")) -> (w1067:string)
            n271 = Search and Replace String(input string=w1069, search string="[<C>]", replace string=w1067) -> (result string=w1066:string)  [unwired: 5 in, 3 out]
            n272 = Search and Replace String(input string=w1070, search string=w1067, replace string=w1066) -> (result string=w1065:string)  [unwired: 5 in, 3 out]
          }
        }
      }
      "CASTed String" <- w973
      n273 = call "DB - Replace DB.Schema.Table.vi"("DB.Schema.Table 3"=w988, "DB.Schema.Table 2"=w1049, "DB.Schema.Table"=w1054, "string in"=w973) -> ("error out"=w1012:errorcluster, "string out"=w1051:string)  [unwired: 6 in]
      n274 = Search and Replace String(input string=w1051, search string="<A>", replace string=w1011, error in=w1012) -> (result string=w998:string)  [unwired: 4 in, 3 out]
      n275 = Search and Replace String(input string=w998, search string="<CONDITION1>", replace string=w995) -> (result string=w997:string)  [unwired: 5 in, 3 out]
      n276 = Search and Replace String(input string=w997, search string="<CONDITION2>", replace string=w1006) -> (result string=w1010:string)  [unwired: 5 in, 3 out]
      n277 = call-poly <vilib>:"DB Tools Execute Query.vi"("SQL query"=w1010, "connection reference"=w1053) -> ("error out"=w1060:errorcluster, "recordset reference"=w1059:T20)  [unwired: 6 in]
      n278 = call-poly <vilib>:"DB Tools Fetch Recordset Data.vi"("error in (no error)"=w1060, "recordset reference"=w1059) -> ("error out"=w1055:errorcluster, "recordset data"=w1058:variant[][], "recordset reference out"=w1056:T20)  [unwired: 3 in]
      n279 = xnode "Database Variant To Data"("database variant"=w1058, "type"=string[][] []) -> ("data"=w985:string[][], "error out"=w979:errorcluster)  [unwired: 1 in]
      n280 = call-poly <vilib>:"DB Tools Free Object.vi"("error in (no error)"=w1055, "recordset reference"=w1056) -> ("error out"=w1013:errorcluster, "connection reference"=w1052:T14)  [unwired: 8 in]
      n281 = Index Array(array=w985, index (row)=0) -> (element=w984:string[])  [unwired: 1 in]
      n282 = Index Array(array=w984, index #1=DB_-_[TransactionNo],[OrderNo]."h.[ProcedureNo]" ("h.[TransactionNo],i.[OrderNo]\n2014-09-27 11:16"), index #3=DB_-_[TransactionNo],[OrderNo]."h.[HoldTemperature]" ("h.[TransactionNo],i.[OrderNo]\n2014-09-27 11:16")) -> (element #1=w1043:string, element #2=w1042:string, element #3=w1041:string, element #4=w1040:string, element #5=w1039:string)  [unwired: 3 in]
      n283 = Index Array(array=w984, index #1=DB_-_[TransactionNo],[OrderNo]."h.[WPSNo]" ("h.[TransactionNo],i.[OrderNo]\n2014-09-27 11:16")) -> (element #1=w1037:string, element #2=w1035:string)  [unwired: 1 in]
      n284 = Array Subset(array=w985, index (row)=w1030, index (col)=DB_-_[TransactionNo],[OrderNo]."i.[itemNo]" ("h.[TransactionNo],i.[OrderNo]\n2014-09-27 11:16")) -> (w1029:string[][])  [unwired: 2 in]
      n285 = Index Array(array=w984, index=DB_-_[TransactionNo],[OrderNo]."h.[AdditionalProcs]" ("h.[TransactionNo],i.[OrderNo]\n2014-09-27 11:16")) -> (element=w1023:string)
      n286 = Index Array(array=w984, index #1=DB_-_[TransactionNo],[OrderNo]."h.[OutputSetId]" ("h.[TransactionNo],i.[OrderNo]\n2014-09-27 11:16"), index #2=DB_-_[TransactionNo],[OrderNo]."j.[Description]" ("h.[TransactionNo],i.[OrderNo]\n2014-09-27 11:16")) -> (element #1=w982:string, element #2=w981:string)
      n287 = Bundle By Name(cluster=T9 {"WPS/Ref"="WPS5", "Rev"="1", "Hold Temperature"="100", "WPS Details Temperature Units"="°C", "Hold Time (HH:MM)"="1:00", "Inactive"=FALSE} ("WPS Details Setup"), "WPS/Ref"=w1043, "Rev"=w1042, "Hold Temperature"=w1041, "WPS Details Temperature Units"=w1040, "Hold Time (HH:MM)"=w1039) -> (w1044:T9)
      n288 = Spreadsheet String To Array(delimiter (Tab)=",", format string="", spreadsheet string=w1023, array type (2D Dbl)=string[][] []) -> (array=w1020:string[][])
      n289 = call "DB - Sort Item Names To DB.vi"("DB Query Array"=w1029) -> ("ItemNames"=w1028:string[][])  [unwired: 9 in, 1 out]
      n290 = for {
        tunnel: w985 -> [w1079] mode=indexing
        tunnel: [w1078] -> w1005 mode=indexing
        n291 = Array To Spreadsheet String(delimiter (Tab)=",", array=w1079, 3:"" ("format string")) -> (spreadsheet string=w1078:string)
      }
      n292 = Bundle(w982, w981) -> (w980:cluster{string, string})  [unwired: 1 in]
      n293 = call "VI - Interactive or SubVI.vi"() -> ("Mode"=w987:T16)  [unwired: 5 in]
      n294 = property on="MCListBox AWPS" class="MCListbox (strict)"(error in=w979, "ItemNames"=w1020) -> (error out=w1015:errorcluster)  [unwired: 1 in, 1 out]
      n295 = property on="WPS Details Setup" class="Clust (strict)"(error in=w979, "Value"=w1044) -> (error out=w1018:errorcluster)  [unwired: 1 in, 1 out]
      n296 = property on="Extra WPS" class="Str"(error in=w979, "Value"=w1037) -> (error out=w1017:errorcluster)  [unwired: 1 in, 1 out]
      n297 = property on="Extra Rev" class="Str"(error in=w979, "Value"=w1035) -> (error out=w1016:errorcluster)  [unwired: 1 in, 1 out]
      n298 = property on="Part Details" class="MCListbox (strict)"(error in=w979, "ItemNames"=w1028) -> (error out=w1014:errorcluster)  [unwired: 1 in, 1 out]
      n299 = property on="Results Output" class="Clust (strict)"(error in=w979, "Value"=w980) -> (error out=w978:errorcluster)  [unwired: 1 in, 1 out]
      n300 = case shown="\"subVI Mode\"" w987 {
        tunnel: w986 -> [_ w1077]
        tunnel: w980 -> [_ w1076]
        tunnel: [_ w1075] -> w977
        tunnel: w978 -> [_ w1074]
        frame "Interactive", Default {
        }
        frame "subVI Mode" {
          n301 = property class="Clust (strict)"(reference=w1077, error in=w1074, "Value"=w1076) -> (error out=w1075:errorcluster)  [unwired: 1 out]
        }
      }
      n302 = case shown="\"subVI Mode\"" w987 {
        tunnel: w1045 -> [_ w1101]
        tunnel: w1044 -> [_ w1100]
        tunnel: [_ w1099] -> w1034
        tunnel: w1018 -> [_ w1098]
        frame "Interactive", Default {
        }
        frame "subVI Mode" {
          n303 = property class="Clust (strict)"(reference=w1101, error in=w1098, "Value"=w1100) -> (error out=w1099:errorcluster)  [unwired: 1 out]
        }
      }
      n304 = case shown="\"subVI Mode\"" w987 {
        tunnel: w1038 -> [_ w1097]
        tunnel: w1037 -> [_ w1096]
        tunnel: [_ w1095] -> w1033
        tunnel: w1017 -> [_ w1094]
        frame "Interactive", Default {
        }
        frame "subVI Mode" {
          n305 = property class="Str"(reference=w1097, error in=w1094, "Value"=w1096) -> (error out=w1095:errorcluster)  [unwired: 1 out]
        }
      }
      n306 = case shown="\"subVI Mode\"" w987 {
        tunnel: w1036 -> [_ w1093]
        tunnel: w1035 -> [_ w1092]
        tunnel: [_ w1091] -> w1032
        tunnel: w1016 -> [_ w1090]
        frame "Interactive", Default {
        }
        frame "subVI Mode" {
          n307 = property class="Str"(reference=w1093, error in=w1090, "Value"=w1092) -> (error out=w1091:errorcluster)  [unwired: 1 out]
        }
      }
      n308 = case shown="\"subVI Mode\"" w987 {
        tunnel: w1024 -> [_ w1085]
        tunnel: w1020 -> [_ w1084]
        tunnel: [_ w1083] -> w1025
        tunnel: w1015 -> [_ w1082]
        frame "Interactive", Default {
        }
        frame "subVI Mode" {
          n309 = property class="MCListbox (strict)"(reference=w1085, error in=w1082, "ItemNames"=w1084) -> (error out=w1083:errorcluster)  [unwired: 1 out]
        }
      }
      n310 = case shown="\"subVI Mode\"" w987 {
        tunnel: w1027 -> [_ w1089]
        tunnel: w1028 -> [_ w1088]
        tunnel: [_ w1087] -> w1026
        tunnel: w1014 -> [_ w1086]
        frame "Interactive", Default {
        }
        frame "subVI Mode" {
          n311 = property class="MCListbox (strict)"(reference=w1089, error in=w1086, "ItemNames"=w1088) -> (error out=w1087:errorcluster)  [unwired: 1 out]
        }
      }
      n312 = Merge Errors(w1034, w1033, w1032, w1025, w1026, w977) -> (w1031:errorcluster)
      n313 = local write "Refnums error out"(w1031) -> ()
    }
  }
  "SUMMARY" <- w23
  "connection reference" <- w58
  "1D Results" <- w61
  "SQL 2D" <- w38
  "2D Results" <- w37
  "Spreadsheet String" <- w24
  "SQL 1D Array" <- w59
  n314 = flat-sequence {
    tunnel: [w1146] -> w62
    frame #0 {
      n315 = Tick Count (ms)() -> (millisecond timer value=w1146:u32)
    }
  }
  n316 = flat-sequence {
    tunnel: w62 -> [w1148]
    frame #0 {
      n317 = Tick Count (ms)() -> (millisecond timer value=w1149:u32)
      n318 = Subtract(x=w1149, y=w1148) -> (x-y=→"ms":u32)
    }
  }
  n319 = Bundle("TransactionNo"=w27, "TransactionRunNo"=w25) -> (→"Transaction":T23)  [unwired: 1 in]
  n320 = case shown="True" w55 {
    tunnel: w23 -> [_ w1151]
    tunnel: w58 -> [_ w1152]
    frame False {
    }
    frame True {
      n321 = call <vilib>:"DB Tools Close Connection.vi"("error in (no error)"=w1151, "connection reference"=w1152) -> ("error out"=→"Close Error":errorcluster)  [unwired: 5 in]
    }
  }
  n322 = global write "Global SRTRS.vi" "DB Error"(w23) -> ()
